vi "PPMS_Data_Recorder.vi"() -> ()   [LabVIEW 2021]
uses:
  <instrlib>/Stanford Research 830/Public/Data/Read (All Parameters).vi
  <instrlib>/Keithley 24XX/Public/Data/Read (Single Point).vi
  <instrlib>/Keithley 24XX/Keithley 24XX.lvlib
  <instrlib>/Stanford Research 830/Stanford Research 830.lvlib
panel:
  out "Phase-Vg":cluster{dbl[], dbl[]}[](graph)
  out "Leak-Vg":cluster{dbl[], dbl[]}[](graph)
  out "Signal-T":cluster{dbl[], dbl[]}[](graph)
  out "Signal-B":cluster{dbl[], dbl[]}[](graph)
  out "Signal-Vg":cluster{dbl[], dbl[]}[](graph)
  out "Voltage #3":sgl
  out "Leakage Current #3":sgl
  out "X-Value 3":dbl
  out "Theta-Value 3":dbl
  out "R-Value 3":dbl
  in  "Keithley #3 Ramp":bool
  in  "Keith#3 Comp. Lvl":dbl=1e-07
  in  "System #3 Enabled/Disabled":bool
  in  "Keithley #3":refnum<visa-resource-name>
  in  "SR830 #3":refnum<visa-resource-name>="GPIB0::10::INSTR"
  in  "SR830 #3 Input Connection":u16(ring) items=["Single-Ended Voltage", "Differential Voltage", "1 MOhm Current Gain", "100 MOhm Current Gain"]
  in  "SR830 #3\nInput Coupling":u16(ring) items=["AC", "DC"]
  in  "SR830 #3 Input \nShield Grounding":u16(ring) items=["Float", "Ground"]
  in  "SR830 #3 Input\nNotch Filter":u16(ring) items=["None", "Line Notch", "2x Line Notch", "Both Notch Filters"]
  in  "SR830 #3 Trigger Source":u16(ring) items=["Internal", "External"]
  in  "SR830 #3 Internal \nReference Frequency":dbl=17.0
  in  "SR830 #3 Detection Harm. Num.":dbl=1.0
  in  "SR830 #3 Sine \nOutput Amplitude":dbl=1.0
  in  "SR830 #3 Reference Source":u16(ring)=1 items=["External", "Internal"]
  in  "SR830 #3 Manual \nPhase":dbl
  in  "SR830 #3 \nAuto Phase":bool
  in  "SR830 #3 \nTime Constant":u16(ring)=9 items=["10 us", "30 us", "100 us", "300 us", "1 ms", "3 ms", "10 ms", "30 ms", "100 ms", "300 ms", "1 s", "3 s", "10 s", "30 s", "100 s", "300 s", "1 ks", "3 ks", "10 ks", "30 ks"]
  in  "SR830 #3 Low\nPass Filter Slope":u16(ring)=3 items=["6 dB/oct", "12 dB/oct", "18 db/oct", "24 dB/oct"]
  in  "SR830 #3\nSync Filter":bool
  in  "SR830 #3 \nDynamic Reserve":i16(ring)=1 items=["Auto Reserve"=-1, "High Reserve"=0, "Normal"=1, "Low Noise"=2]
  in  "SR830 #3\nSensitivity":i16(ring)=17 items=["Auto Gain"=-1, "2 nV/fA"=0, "5 nV/fA"=1, "10 nV/fA"=2, "20 nV/fA"=3, "50 nV/fA"=4, "100 nV/fA"=5, "200 nV/fA"=6, "500 nV/fA"=7, "1 uV/pA"=8, "2 uV/pA"=9, "5 uV/pA"=10, "10 uV/pA"=11, "20 uV/pA"=12, "50 uV/pA"=13, "100 uV/pA"=14, "200 uV/pA"=15, "500 uV/pA"=16, "1 mV/nA"=17, "2 mV/nA"=18, "5 mV/nA"=19, "10 mV/nA"=20, "20 mV/nA"=21, "50 mV/nA"=22, "100 mV/nA"=23, "200 mV/nA"=24, "500 mV/mA"=25, "1 V/uA"=26]
  in  "Keithley #3 Vg Init. (V)":dbl
  in  "Keithley #3 Vg Max (V)":dbl
  in  "Keithley #3 Vg Min (V)":dbl
  in  "Keithley #3 Vg Step (V)":dbl
  out "Voltage #2":sgl
  out "Leakage Current #2":sgl
  out "X-Value 2":dbl
  out "Theta-Value 2":dbl
  out "R-Value 2":dbl
  in  "Keithley #2 Ramp":bool
  in  "Keith#2 Comp. Lvl":dbl=1e-07
  in  "System #2 Enabled/Disabled":bool
  in  "Keithley #2":refnum<visa-resource-name>
  in  "SR830 #2":refnum<visa-resource-name>="GPIB0::10::INSTR"
  in  "SR830 #2 Input Connection":u16(ring) items=["Single-Ended Voltage", "Differential Voltage", "1 MOhm Current Gain", "100 MOhm Current Gain"]
  in  "SR830 #2\nInput Coupling":u16(ring) items=["AC", "DC"]
  in  "SR830 #2 Input \nShield Grounding":u16(ring) items=["Float", "Ground"]
  in  "SR830 #2 Input\nNotch Filter":u16(ring) items=["None", "Line Notch", "2x Line Notch", "Both Notch Filters"]
  in  "SR830 #2 Trigger Source":u16(ring) items=["Internal", "External"]
  in  "SR830 #2 Internal \nReference Frequency":dbl=17.0
  in  "SR830 #2 Detection Harm. Num.":dbl=1.0
  in  "SR830 #2 Sine \nOutput Amplitude":dbl=1.0
  in  "SR830 #2 Reference Source":u16(ring)=1 items=["External", "Internal"]
  in  "SR830 #2 Manual \nPhase":dbl
  in  "SR830 #2 \nAuto Phase":bool
  in  "SR830 #2 \nTime Constant":u16(ring)=9 items=["10 us", "30 us", "100 us", "300 us", "1 ms", "3 ms", "10 ms", "30 ms", "100 ms", "300 ms", "1 s", "3 s", "10 s", "30 s", "100 s", "300 s", "1 ks", "3 ks", "10 ks", "30 ks"]
  in  "SR830 #2 Low\nPass Filter Slope":u16(ring)=3 items=["6 dB/oct", "12 dB/oct", "18 db/oct", "24 dB/oct"]
  in  "SR830 #2\nSync Filter":bool
  in  "SR830 #2 \nDynamic Reserve":i16(ring)=1 items=["Auto Reserve"=-1, "High Reserve"=0, "Normal"=1, "Low Noise"=2]
  in  "SR830 #2\nSensitivity":i16(ring)=17 items=["Auto Gain"=-1, "2 nV/fA"=0, "5 nV/fA"=1, "10 nV/fA"=2, "20 nV/fA"=3, "50 nV/fA"=4, "100 nV/fA"=5, "200 nV/fA"=6, "500 nV/fA"=7, "1 uV/pA"=8, "2 uV/pA"=9, "5 uV/pA"=10, "10 uV/pA"=11, "20 uV/pA"=12, "50 uV/pA"=13, "100 uV/pA"=14, "200 uV/pA"=15, "500 uV/pA"=16, "1 mV/nA"=17, "2 mV/nA"=18, "5 mV/nA"=19, "10 mV/nA"=20, "20 mV/nA"=21, "50 mV/nA"=22, "100 mV/nA"=23, "200 mV/nA"=24, "500 mV/mA"=25, "1 V/uA"=26]
  in  "Keithley #2 Vg Init. (V)":dbl
  in  "Keithley #2 Vg Max (V)":dbl
  in  "Keithley #2 Vg Min (V)":dbl
  in  "Keithley #2 Vg Step (V)":dbl
  out "Temperature":dbl
  out "Field":dbl
  in  "Remote":bool
  out "Chamber Status":i32(ring) items=["ChamberUnknown"=0, "PurgedAndSealed"=1, "VentedAndSealed"=2, "Sealed"=3, "Purging"=4, "Venting"=5, "PreHiVac"=6, "HighVac"=7, "PumpContinuous"=8, "VentContinuous"=9, "ChamberFailure"=15]
  out "Measuring":bool
  out "R-Value":dbl
  out "Theta-Value":dbl
  out "X-Value":dbl
  out "Leakage Current #1":sgl
  out "Voltage #1":sgl
  in  "Keithley #1 Ramp":bool
  in  "Keith#1 Comp. Lvl":dbl=1e-07
  in  "Keithley #1 Vg Step (V)":dbl
  in  "Keithley #1 Vg Max (V)":dbl
  in  "Keithley #1 Vg Min (V)":dbl
  in  "Keithley #1 Vg Init. (V)":dbl
  in  "Keithley #1":refnum<visa-resource-name>
  in  "SR830 #1\nSensitivity":i16(ring)=17 items=["Auto Gain"=-1, "2 nV/fA"=0, "5 nV/fA"=1, "10 nV/fA"=2, "20 nV/fA"=3, "50 nV/fA"=4, "100 nV/fA"=5, "200 nV/fA"=6, "500 nV/fA"=7, "1 uV/pA"=8, "2 uV/pA"=9, "5 uV/pA"=10, "10 uV/pA"=11, "20 uV/pA"=12, "50 uV/pA"=13, "100 uV/pA"=14, "200 uV/pA"=15, "500 uV/pA"=16, "1 mV/nA"=17, "2 mV/nA"=18, "5 mV/nA"=19, "10 mV/nA"=20, "20 mV/nA"=21, "50 mV/nA"=22, "100 mV/nA"=23, "200 mV/nA"=24, "500 mV/mA"=25, "1 V/uA"=26]
  in  "SR830 #1 \nDynamic Reserve":i16(ring)=1 items=["Auto Reserve"=-1, "High Reserve"=0, "Normal"=1, "Low Noise"=2]
  in  "SR830 #1\nSync Filter":bool
  in  "SR830 #1 Low\nPass Filter Slope":u16(ring)=3 items=["6 dB/oct", "12 dB/oct", "18 db/oct", "24 dB/oct"]
  in  "SR830 #1 \nTime Constant":u16(ring)=8 items=["10 us", "30 us", "100 us", "300 us", "1 ms", "3 ms", "10 ms", "30 ms", "100 ms", "300 ms", "1 s", "3 s", "10 s", "30 s", "100 s", "300 s", "1 ks", "3 ks", "10 ks", "30 ks"]
  in  "SR830 #1 \nAuto Phase":bool
  in  "SR830 #1 Manual \nPhase":dbl
  in  "SR830 #1 Reference Source":u16(ring)=1 items=["External", "Internal"]
  in  "SR830 #1 Sine \nOutput Amplitude":dbl=1.0
  in  "SR830 #1 Detection Harm. Num.":dbl=1.0
  in  "SR830 #1 Internal \nReference Frequency":dbl=17.0
  in  "SR830 #1 Trigger Source":u16(ring) items=["Internal", "External"]
  in  "SR830 #1 Input\nNotch Filter":u16(ring) items=["None", "Line Notch", "2x Line Notch", "Both Notch Filters"]
  in  "SR830 #1 Input \nShield Grounding":u16(ring) items=["Float", "Ground"]
  in  "SR830 #1\nInput Coupling":u16(ring) items=["AC", "DC"]
  in  "SR830 #1 Input Connection":u16(ring) items=["Single-Ended Voltage", "Differential Voltage", "1 MOhm Current Gain", "100 MOhm Current Gain"]
  in  "SR830 #1":refnum<visa-resource-name>="GPIB0::10::INSTR"
  in  "System #1 Enabled/Disabled":bool
  in  "System Reset All?":bool
  in  "program_stop":bool
  out "Actual Save Path":path
  in  "<File Name>.txt (Don't add extension)":string
  in  "Data Save Path:":path=path "C:/Users/labpc/Documents/ProbeStation Users Data"
  # "Readout (Recorded)"
  # "Keithley 24XX"
  # "Ramp Settings"
  # "Current Compliance"
  # "SR830"
  # "Input Signal"
  # "Readout (Recorded)"
  # "Source / Reference"
  # "Input Filters & Sens"
  # "Readout (Recorded)"
  # "Keithley 24XX"
  # "Ramp Settings"
  # "Current Compliance"
  # "SR830"
  # "Input Signal"
  # "Readout (Recorded)"
  # "Source / Reference"
  # "Input Filters & Sens"
  # "PPMS"
  # "Readout (Recorded)"
  # "Keithley 24XX"
  # "Ramp Settings"
  # "Current Compliance"
  # "SR830"
  # "Input Signal"
  # "Readout (Recorded)"
  # "Source / Reference"
  # "Input Filters & Sens"
  # "Initialisation:\n--> Reset \n--> Instruments?"
  # "File I/O"
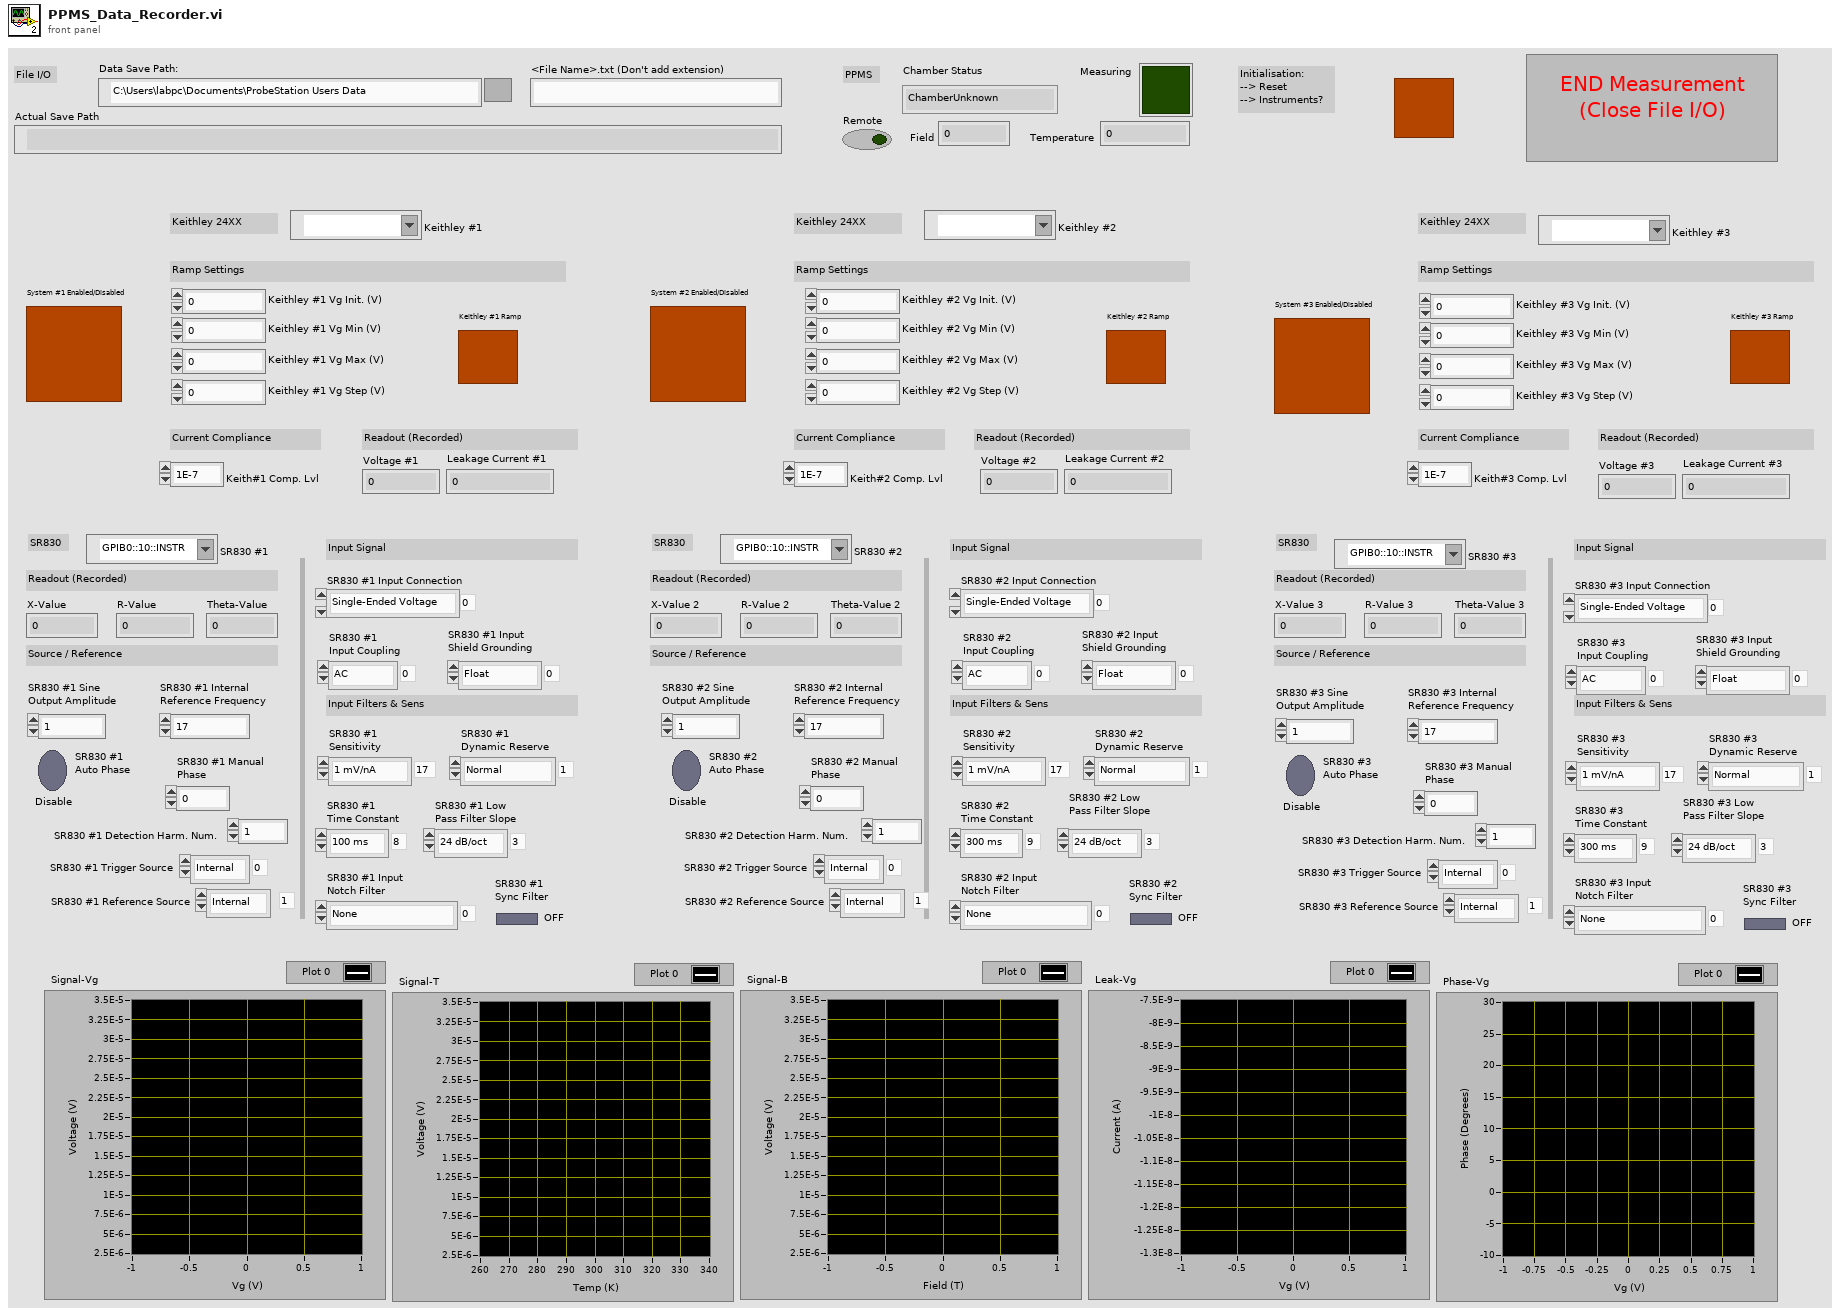
[diagram p1: front panel]
types:
  T1 = enum16{"open", "replace", "create", "open or create", "replace or create", "replace or create with confirmation"}
  T2 = cluster{"System #1 Enabled/Disabled":bool, "System #2 Enabled/Disabled":bool, "System #3 Enabled/Disabled":bool}
  T3 = cluster{"VISA resource name out":refnum<visa-resource-name>, "error out":errorcluster, "VISA resource name out":refnum<visa-resource-name>, "error out":errorcluster, "Keithley #1 Vg Init. (V)":dbl, "Keithley #1 Vg Max (V)":dbl, "Keithley #1 Vg Min (V)":dbl, "Keithley #1 Vg Step (V)":dbl, "Keith#1 Comp. Lvl":dbl}
  T4 = cluster{"Baud Rate":u32, "Parity":u16, "Data Bits":u16, "Stop Bits":u16, "Flow Control":u16}
  T5 = cluster{"VISA resource name out":refnum<visa-resource-name>, "error out":errorcluster, "VISA resource name out":refnum<visa-resource-name>, "error out":errorcluster, "Keithley #2 Vg Init. (V)":dbl, "Keithley #2 Vg Max (V)":dbl, "Keithley #2 Vg Min (V)":dbl, "Keithley #2 Vg Step (V)":dbl, "Keith#2 Comp. Lvl":dbl}
  T6 = cluster{"VISA resource name out":refnum<visa-resource-name>, "error out":errorcluster, "VISA resource name out":refnum<visa-resource-name>, "error out":errorcluster, "Keithley #3 Vg Init. (V)":dbl, "Keithley #3 Vg Max (V)":dbl, "Keithley #3 Vg Min (V)":dbl, "Keithley #3 Vg Step (V)":dbl, "Keith#3 Comp. Lvl":dbl}
  T7 = cluster{"array":dbl[][], "array":dbl[][], "array":dbl[][], "array":dbl[][]}
  T8 = cluster{"Voltage":sgl, "Current":sgl, "X-Value":dbl, "R-Value":dbl, "Theta-Value":dbl}
  T9 = enum8{"Enabled", "Disabled", "Disabled and Grayed Out"}
  T10 = cluster{"X-Value":dbl, "Y-Value":dbl, "R-Value":dbl, "Theta-Value":dbl, "Aux In 1 Value":dbl, "Aux In 2 Value":dbl, "Aux In 3 Value":dbl, "Aux In 4 Value":dbl, "Reference Frequency":dbl, "Channel 1 Display":dbl, "Channel 2 Display":dbl}
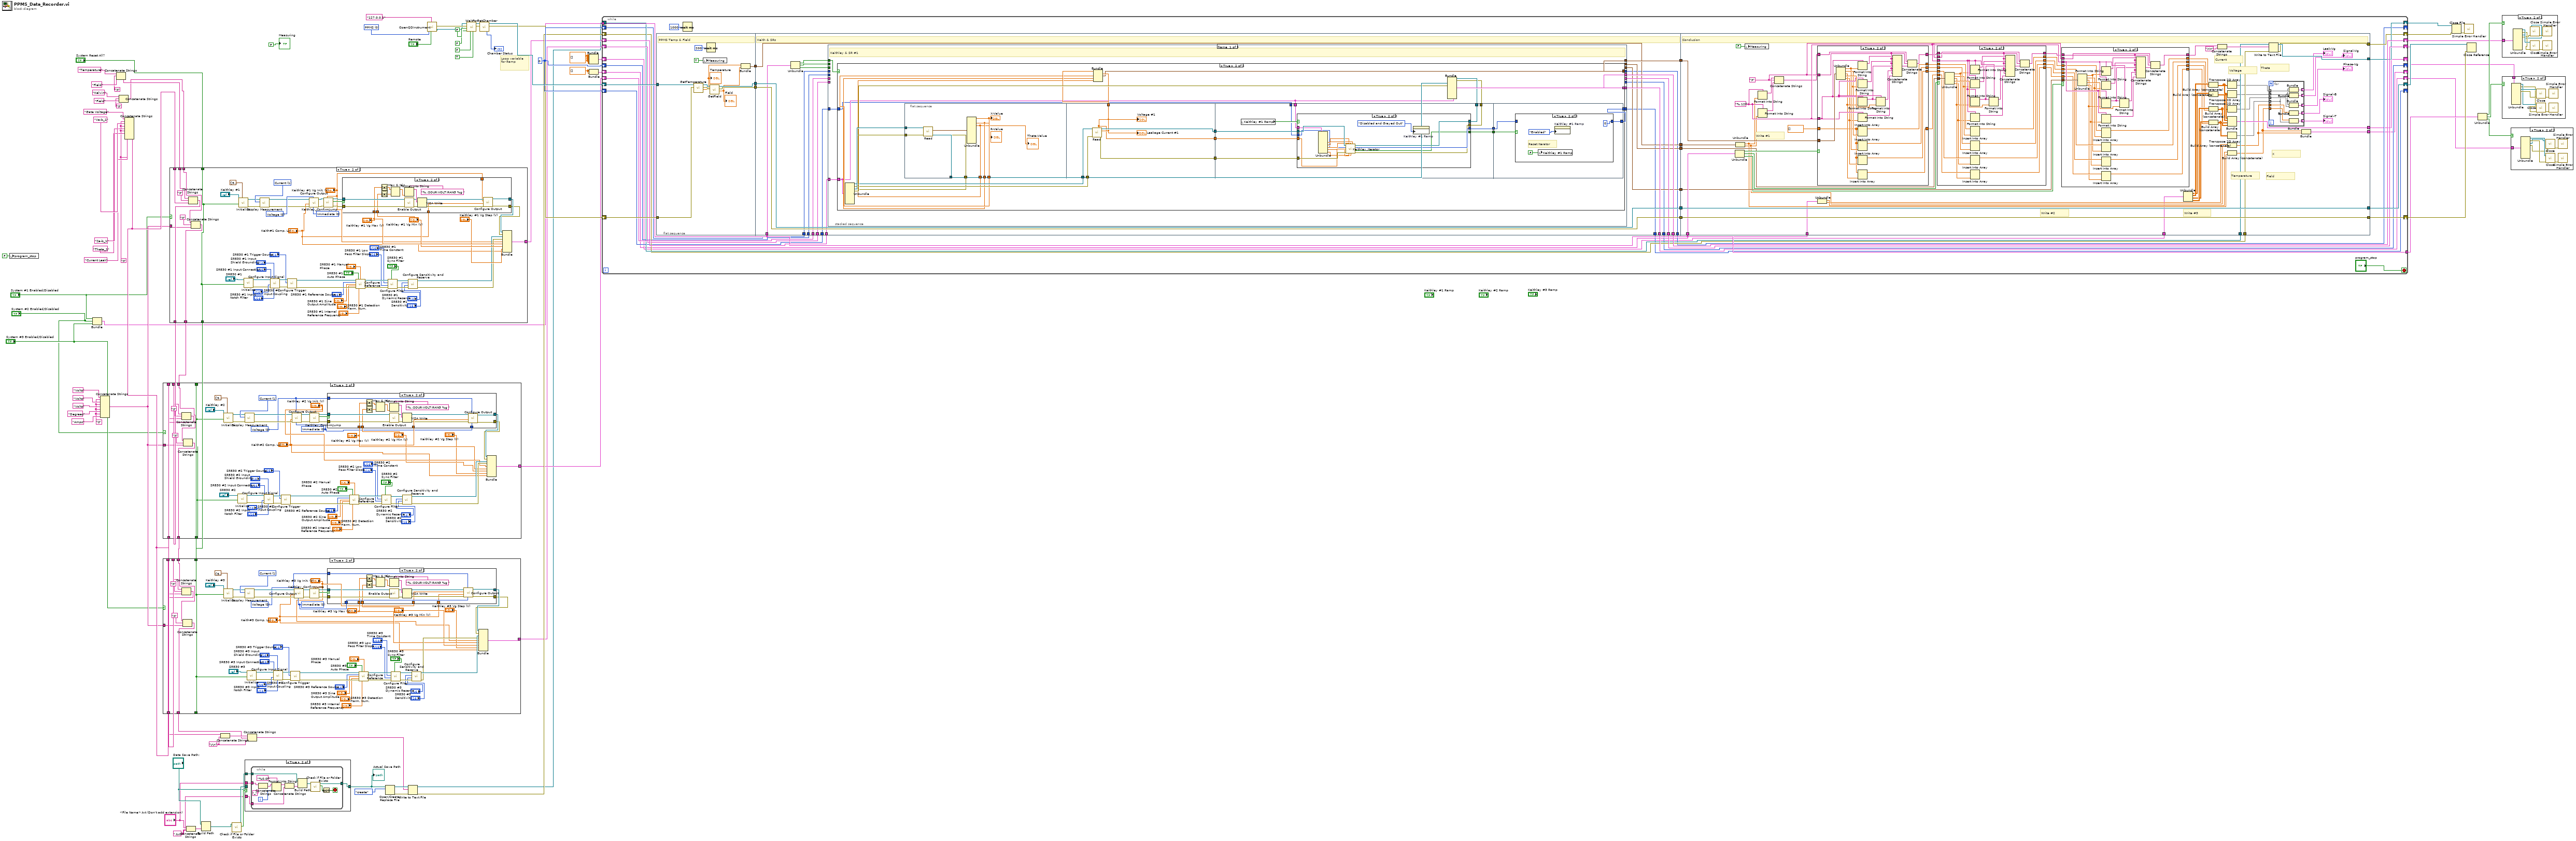
[diagram p0: block diagram]
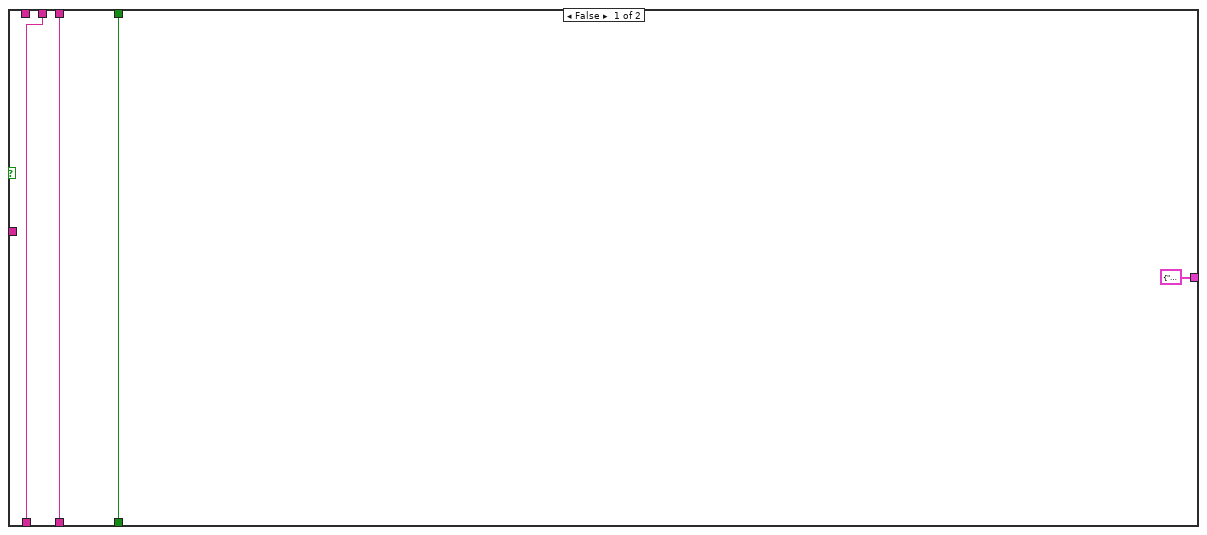
[diagram p5: hidden frame]
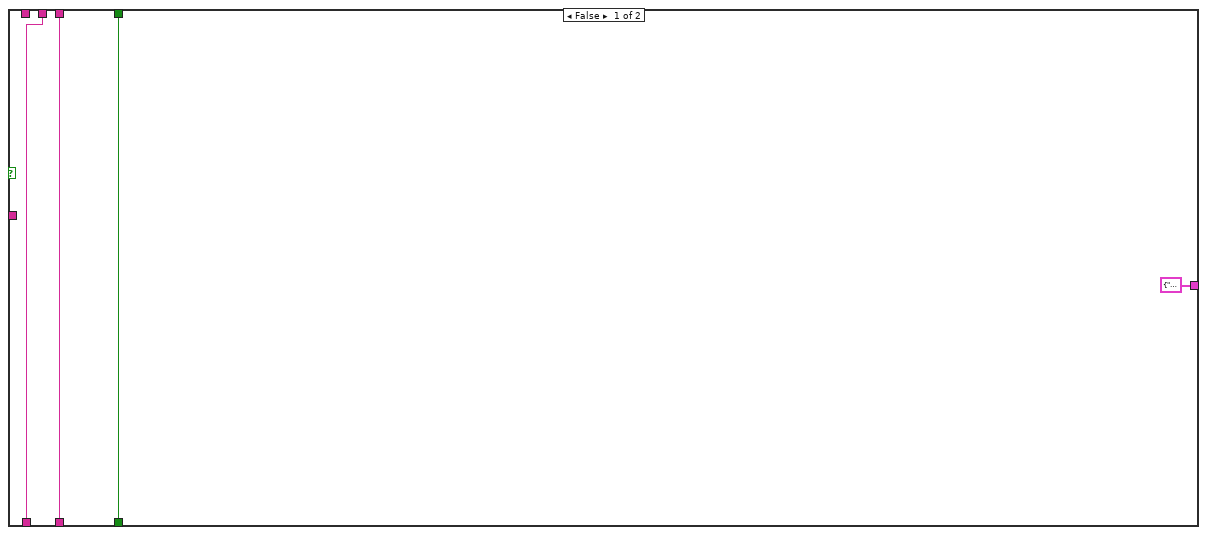
[diagram p7: hidden frame]
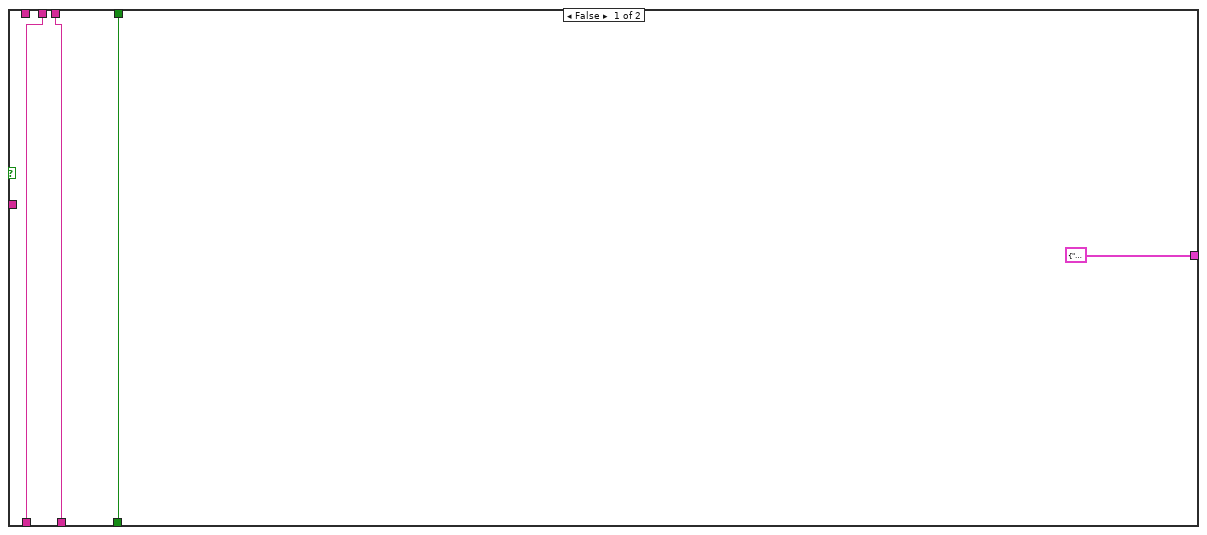
[diagram p9: hidden frame]
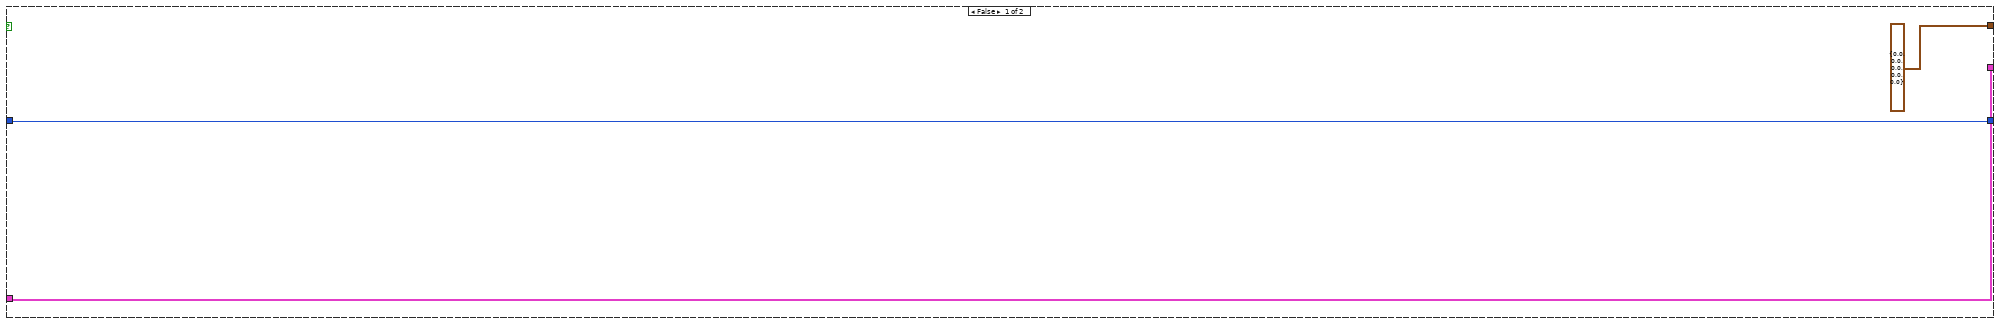
[diagram p12: hidden frame]
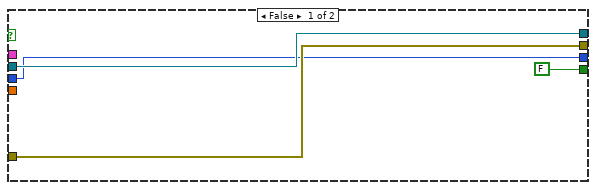
[diagram p13: hidden frame]
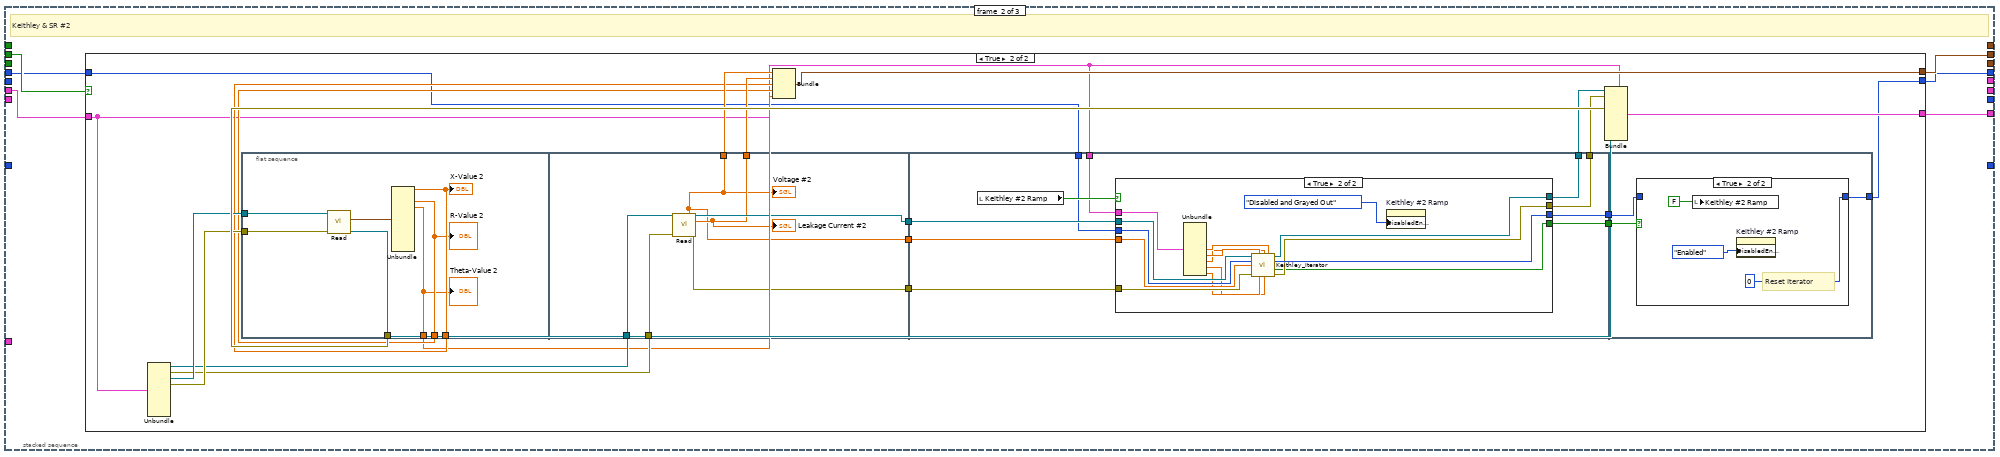
[diagram p15: hidden frame]
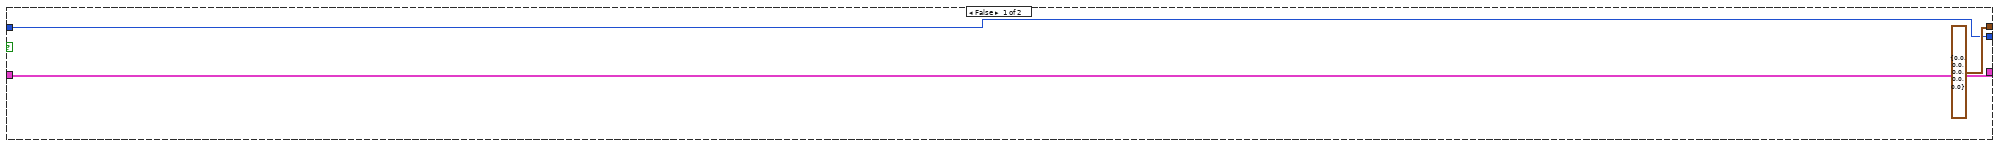
[diagram p16: hidden frame]
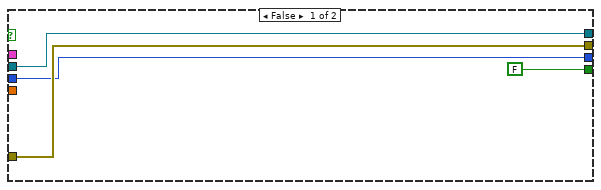
[diagram p17: hidden frame]
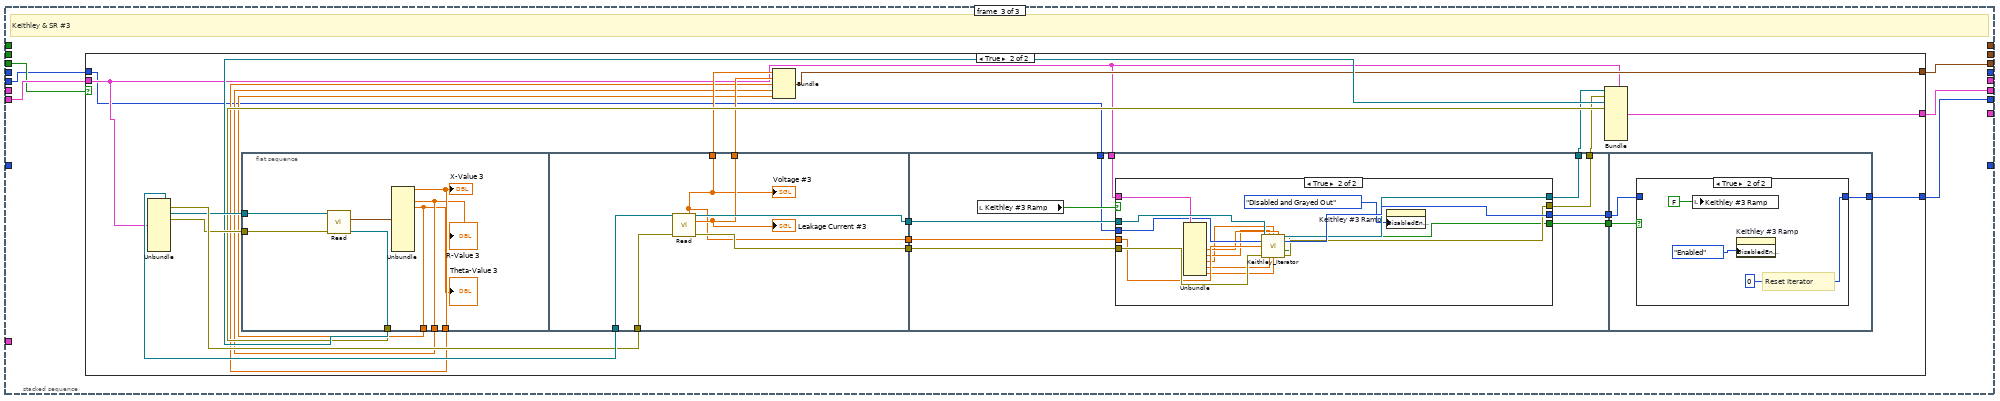
[diagram p19: hidden frame]
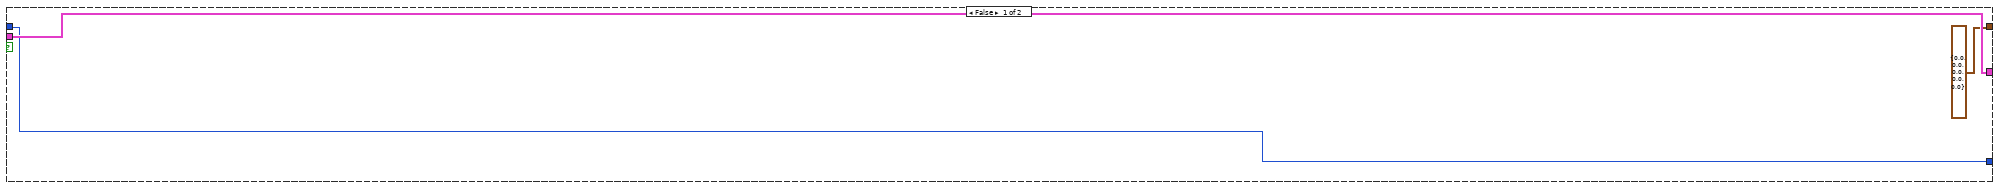
[diagram p20: hidden frame]
diagram:
  w5 = dbl[][] [] ("array")
  w7 = dbl[] [] ("array")
  w29 = 0
  w44 = "\t"
  w33 = "\r\n"
  w58 = "\t"
  w67 = 0 items=["PPMS", "VersaLab", "DynaCool", "SVSM"] ("Instrument Type")
  w70 = ".txt"
  # "Loop variable \nfor Ramp"
  n1 = local write "program_stop"(FALSE ("program_stop")) -> ()
  n2 = Bundle("System #1 Enabled/Disabled"="System #1 Enabled/Disabled", "System #2 Enabled/Disabled"="System #2 Enabled/Disabled", "System #3 Enabled/Disabled"="System #3 Enabled/Disabled") -> (w14:T2)  [unwired: 1 in]
  n3 = Concatenate Strings("Volts" ("string"), w44, "Volts" ("string"), w44, "Volts" ("string"), w44, "Degrees" ("string"), w44, "Amps" ("string")) -> (w36:string)
  n4 = Concatenate Strings("Temperature" ("string"), "\t", "Field" ("string")) -> (w57:string)
  n5 = Concatenate Strings("Kelvin" ("string"), "\t", "Field" ("string")) -> (w39:string)
  n6 = Concatenate Strings("Gate Voltage" ("string"), w58, "Va-b_1" ("string"), w58, "Za-b_1" ("string"), w58, "Theta_1" ("string"), w58, "Current Leak" ("string")) -> (w52:string)
  n7 = case shown="True" "System #1 Enabled/Disabled" {
    tunnel: w52 -> [_ w151]
    tunnel: w57 -> [w91 w149]
    tunnel: [w91 w148] -> w55
    tunnel: "System Reset All?" -> [w90 w106]
    tunnel: [w90 w106] -> w54
    tunnel: w39 -> [w89 w104]
    tunnel: [w89 w103] -> w38
    tunnel: w36 -> [_ w102]
    tunnel: [T3 {"VISA resource name out"="", "error out"={"status"=FALSE, "code"=0, "source"=""}, "VISA resource name out"="", "error out"={"status"=FALSE, "code"=0, "source"=""}, "Keithley #1 Vg Init. (V)"=0.0, "Keithley #1 Vg Max (V)"=0.0, "Keithley #1 Vg Min (V)"=0.0, "Keithley #1 Vg Step (V)"=0.0, "Keith#1 Comp. Lvl"=0.0} w94] -> w20
    frame False {
    }
    frame True {
      w112 = u16 0 items=["Immediate", "Triggered"] ("Output Type  (0: Immediate)")
      w111 = u16 0 items=["Voltage", "Current"] ("Source Mode  (0: Voltage)")
      w146 = u16 1 items=["Voltage", "Current", "Resistance"] ("Displayed Measurement (0: Voltage)")
      n8 = Concatenate Strings(w149, "\t", w151) -> (w148:string)
      n9 = Concatenate Strings(w104, "\t", w102) -> (w103:string)
      n10 = call <instrlib>:"Initialize.vi"("Serial Configuration"=T4 {"Baud Rate"=9600, "Parity"=0, "Data Bits"=8, "Stop Bits"=10, "Flow Control"=0}, "Reset (True)"=w106, "VISA resource name"="Keithley #1") -> ("error out"=w144:errorcluster, "VISA resource name out"=w145:refnum<visa-resource-name>)  [unwired: 7 in]
      n11 = call <instrlib>:"Initialize.vi"("Reset (True)"=w106, "VISA resource name"="SR830 #1") -> ("error out"=w138:errorcluster, "VISA resource name out"=w139:refnum<visa-resource-name>)  [unwired: 8 in]
      n12 = call <instrlib>:"Display Measurement.vi"("error in (no error)"=w144, "Displayed Measurement (0: Voltage)"=w146, "VISA resource name"=w145) -> ("error out"=w109:errorcluster, "VISA resource name out"=w110:refnum<visa-resource-name>)  [unwired: 7 in]
      n13 = call <instrlib>:"Configure Input Signal.vi"("Input Notch Filter (0: None)"="SR830 #1 Input\nNotch Filter", "Input Shield Grounding (0: Float)"="SR830 #1 Input \nShield Grounding", "error in (no error)"=w138, "Input Coupling (0: AC)"="SR830 #1\nInput Coupling", "Input Connection (0: Single-Ended Voltage)"="SR830 #1 Input Connection", "VISA resource name"=w139) -> ("error out"=w136:errorcluster, "VISA resource name out"=w137:refnum<visa-resource-name>)  [unwired: 4 in]
      n14 = call <instrlib>:"Configure Trigger.vi"("error in (no error)"=w136, "Trigger Source (0: Internal)"="SR830 #1 Trigger Source", "VISA resource name"=w137) -> ("error out"=w134:errorcluster, "VISA resource name out"=w135:refnum<visa-resource-name>)  [unwired: 7 in]
      n15 = call <instrlib>:"Configure Output.vi"("Output Type  (0: Immediate)"=w112, "Source Mode  (0: Voltage)"=w111, "error in (no error)"=w109, "Compliance  Level (0.1)"="Keith#1 Comp. Lvl", "VISA resource name"=w110) -> ("error out"=w107:errorcluster, "VISA resource name out"=w108:refnum<visa-resource-name>)  [unwired: 5 in]
      n16 = call "Keithley_ConfirmJump.vi"("VISA resource name in"=w108, "error in"=w107, "Gate Voltage\nInitial (V)"="Keithley #1 Vg Init. (V)") -> ("VISA resource name out"=w114:refnum<visa-resource-name>, "Voltage OK?"=w115:bool, "error out"=w113:errorcluster)  [unwired: 4 in, 1 out]
      n17 = case shown="True" w115 {
        tunnel: w114 -> [w153 w163]
        tunnel: w113 -> [w152 w162]
        tunnel: [w153 w156] -> w98
        tunnel: [w152 w157] -> w97
        tunnel: "Keithley #1 Vg Max (V)" -> [_ w161]
        tunnel: "Keithley #1 Vg Min (V)" -> [_ w160]
        tunnel: "Keithley #1 Vg Init. (V)" -> [_ w155]
        tunnel: "Keith#1 Comp. Lvl" -> [_ w154]
        frame False {
        }
        frame True {
          n18 = Absolute Value(x=w161) -> (abs(x)=w165:dbl)
          n19 = Absolute Value(x=w160) -> (abs(x)=w166:dbl)
          n20 = Max & Min(x=w165, y=w166) -> (max(x,y)=w170:dbl)  [unwired: 1 out]
          n21 = Format Into String(format string="%.;SOUR:VOLT:RANG %g ", w170) -> (resulting string=w169:string)  [unwired: 2 in, 1 out]
          n22 = call <instrlib>:"Enable Output.vi"("error in (no error)"=w162, "VISA resource name"=w163) -> ("error out"=w167:errorcluster, "VISA resource name out"=w168:refnum<visa-resource-name>)  [unwired: 8 in]
          n23 = VISA Write(VISA resource name=w168, write buffer=w169, error in (no error)=w167) -> (VISA resource name out=w159:refnum<visa-resource-name>, error out=w158:errorcluster)  [unwired: 1 out]
          n24 = call <instrlib>:"Configure Output.vi"("error in (no error)"=w158, "Compliance  Level (0.1)"=w154, "Output Level (0)"=w155, "VISA resource name"=w159) -> ("error out"=w157:errorcluster, "VISA resource name out"=w156:refnum<visa-resource-name>)  [unwired: 6 in]
        }
      }
      n25 = call <instrlib>:"Configure Reference.vi"("VISA resource name"=w135, "Auto Phase (T: Enabled)"="SR830 #1 \nAuto Phase", "Manual Phase (0 Degree)"="SR830 #1 Manual \nPhase", "Reference Source (1: Internal)"="SR830 #1 Reference Source", "Sine Output Amplitude (1 V)"="SR830 #1 Sine \nOutput Amplitude", "Detection Harmonic Number (1)"="SR830 #1 Detection Harm. Num.", "error in (no error)"=w134, "Internal Reference Frequency (1000 Hz)"="SR830 #1 Internal \nReference Frequency") -> ("VISA resource name out"=w132:refnum<visa-resource-name>, "error out"=w133:errorcluster)  [unwired: 6 in]
      n26 = call <instrlib>:"Configure Filter.vi"("Enable Sync Filter (F: Disable)"="SR830 #1\nSync Filter", "error in (no error)"=w133, "Low Pass Filter Slope (1: 12dB/oct)"="SR830 #1 Low\nPass Filter Slope", "Time Constant (8: 100ms)"="SR830 #1 \nTime Constant", "VISA resource name"=w132) -> ("error out"=w118:errorcluster, "VISA resource name out"=w119:refnum<visa-resource-name>)  [unwired: 5 in]
      n27 = call <instrlib>:"Configure Sensitivity and Reserve.vi"("error in (no error)"=w118, "Sensitivity (-1: Auto gain)"="SR830 #1\nSensitivity", "Dynamic Reserve (-1: Auto Reserve)"="SR830 #1 \nDynamic Reserve", "VISA resource name"=w119) -> ("error out"=w95:errorcluster, "VISA resource name out"=w96:refnum<visa-resource-name>)  [unwired: 6 in]
      n28 = Bundle("VISA resource name out"=w98, "error out"=w97, "VISA resource name out"=w96, "error out"=w95, "Keithley #1 Vg Init. (V)"="Keithley #1 Vg Init. (V)", "Keithley #1 Vg Max (V)"="Keithley #1 Vg Max (V)", "Keithley #1 Vg Min (V)"="Keithley #1 Vg Min (V)", "Keithley #1 Vg Step (V)"="Keithley #1 Vg Step (V)", "Keith#1 Comp. Lvl"="Keith#1 Comp. Lvl") -> (w94:T3)  [unwired: 1 in]
    }
  }
  n29 = case shown="True" "System #2 Enabled/Disabled" {
    tunnel: w52 -> [_ w234]
    tunnel: w55 -> [w174 w232]
    tunnel: [w174 w231] -> w53
    tunnel: w54 -> [w173 w195]
    tunnel: [w173 w195] -> w51
    tunnel: w38 -> [w172 w193]
    tunnel: [w172 w192] -> w37
    tunnel: w36 -> [_ w191]
    tunnel: [T5 {"VISA resource name out"="", "error out"={"status"=FALSE, "code"=0, "source"=""}, "VISA resource name out"="", "error out"={"status"=FALSE, "code"=0, "source"=""}, "Keithley #2 Vg Init. (V)"=0.0, "Keithley #2 Vg Max (V)"=0.0, "Keithley #2 Vg Min (V)"=0.0, "Keithley #2 Vg Step (V)"=0.0, "Keith#2 Comp. Lvl"=0.0} w182] -> w19
    frame False {
    }
    frame True {
      w175 = u16 0 items=["Immediate", "Triggered"] ("Output Type  (0: Immediate)")
      w176 = u16 0 items=["Voltage", "Current"] ("Source Mode  (0: Voltage)")
      w229 = u16 1 items=["Voltage", "Current", "Resistance"] ("Displayed Measurement (0: Voltage)")
      n30 = Concatenate Strings(w232, "\t", w234) -> (w231:string)
      n31 = Concatenate Strings(w193, "\t", w191) -> (w192:string)
      n32 = call <instrlib>:"Initialize.vi"("Serial Configuration"=T4 {"Baud Rate"=9600, "Parity"=0, "Data Bits"=8, "Stop Bits"=10, "Flow Control"=0}, "Reset (True)"=w195, "VISA resource name"="Keithley #2") -> ("error out"=w227:errorcluster, "VISA resource name out"=w228:refnum<visa-resource-name>)  [unwired: 7 in]
      n33 = call <instrlib>:"Initialize.vi"("Reset (True)"=w195, "VISA resource name"="SR830 #2") -> ("error out"=w221:errorcluster, "VISA resource name out"=w222:refnum<visa-resource-name>)  [unwired: 8 in]
      n34 = call <instrlib>:"Display Measurement.vi"("error in (no error)"=w227, "Displayed Measurement (0: Voltage)"=w229, "VISA resource name"=w228) -> ("error out"=w180:errorcluster, "VISA resource name out"=w181:refnum<visa-resource-name>)  [unwired: 7 in]
      n35 = call <instrlib>:"Configure Input Signal.vi"("Input Notch Filter (0: None)"="SR830 #2 Input\nNotch Filter", "Input Shield Grounding (0: Float)"="SR830 #2 Input \nShield Grounding", "error in (no error)"=w221, "Input Coupling (0: AC)"="SR830 #2\nInput Coupling", "Input Connection (0: Single-Ended Voltage)"="SR830 #2 Input Connection", "VISA resource name"=w222) -> ("error out"=w219:errorcluster, "VISA resource name out"=w220:refnum<visa-resource-name>)  [unwired: 4 in]
      n36 = call <instrlib>:"Configure Trigger.vi"("error in (no error)"=w219, "Trigger Source (0: Internal)"="SR830 #2 Trigger Source", "VISA resource name"=w220) -> ("error out"=w217:errorcluster, "VISA resource name out"=w218:refnum<visa-resource-name>)  [unwired: 7 in]
      n37 = call <instrlib>:"Configure Output.vi"("Output Type  (0: Immediate)"=w175, "Source Mode  (0: Voltage)"=w176, "error in (no error)"=w180, "Compliance  Level (0.1)"="Keith#2 Comp. Lvl", "VISA resource name"=w181) -> ("error out"=w178:errorcluster, "VISA resource name out"=w177:refnum<visa-resource-name>)  [unwired: 5 in]
      n38 = call "Keithley_ConfirmJump.vi"("VISA resource name in"=w177, "error in"=w178, "Gate Voltage\nInitial (V)"="Keithley #2 Vg Init. (V)") -> ("VISA resource name out"=w197:refnum<visa-resource-name>, "Voltage OK?"=w198:bool, "error out"=w196:errorcluster)  [unwired: 4 in, 1 out]
      n39 = case shown="True" w198 {
        tunnel: w197 -> [w236 w247]
        tunnel: w196 -> [w235 w246]
        tunnel: [w236 w238] -> w190
        tunnel: [w235 w237] -> w189
        tunnel: "Keithley #2 Vg Max (V)" -> [_ w245]
        tunnel: "Keithley #2 Vg Min (V)" -> [_ w244]
        tunnel: w175 -> [_ w243]
        tunnel: w176 -> [_ w242]
        tunnel: "Keith#2 Comp. Lvl" -> [_ w241]
        frame False {
        }
        frame True {
          n40 = Absolute Value(x=w245) -> (abs(x)=w249:dbl)
          n41 = Absolute Value(x=w244) -> (abs(x)=w250:dbl)
          n42 = Max & Min(x=w249, y=w250) -> (max(x,y)=w254:dbl)  [unwired: 1 out]
          n43 = Format Into String(format string="%.;SOUR:VOLT:RANG %g ", w254) -> (resulting string=w253:string)  [unwired: 2 in, 1 out]
          n44 = call <instrlib>:"Enable Output.vi"("error in (no error)"=w246, "VISA resource name"=w247) -> ("error out"=w251:errorcluster, "VISA resource name out"=w252:refnum<visa-resource-name>)  [unwired: 8 in]
          n45 = VISA Write(VISA resource name=w252, write buffer=w253, error in (no error)=w251) -> (VISA resource name out=w240:refnum<visa-resource-name>, error out=w239:errorcluster)  [unwired: 1 out]
          n46 = call <instrlib>:"Configure Output.vi"("Output Type  (0: Immediate)"=w243, "Source Mode  (0: Voltage)"=w242, "error in (no error)"=w239, "Compliance  Level (0.1)"=w241, "VISA resource name"=w240) -> ("error out"=w237:errorcluster, "VISA resource name out"=w238:refnum<visa-resource-name>)  [unwired: 5 in]
        }
      }
      n47 = call <instrlib>:"Configure Reference.vi"("VISA resource name"=w218, "Auto Phase (T: Enabled)"="SR830 #2 \nAuto Phase", "Manual Phase (0 Degree)"="SR830 #2 Manual \nPhase", "Reference Source (1: Internal)"="SR830 #2 Reference Source", "Sine Output Amplitude (1 V)"="SR830 #2 Sine \nOutput Amplitude", "Detection Harmonic Number (1)"="SR830 #2 Detection Harm. Num.", "error in (no error)"=w217, "Internal Reference Frequency (1000 Hz)"="SR830 #2 Internal \nReference Frequency") -> ("VISA resource name out"=w215:refnum<visa-resource-name>, "error out"=w216:errorcluster)  [unwired: 6 in]
      n48 = call <instrlib>:"Configure Filter.vi"("Enable Sync Filter (F: Disable)"="SR830 #2\nSync Filter", "error in (no error)"=w216, "Low Pass Filter Slope (1: 12dB/oct)"="SR830 #2 Low\nPass Filter Slope", "Time Constant (8: 100ms)"="SR830 #2 \nTime Constant", "VISA resource name"=w215) -> ("error out"=w201:errorcluster, "VISA resource name out"=w202:refnum<visa-resource-name>)  [unwired: 5 in]
      n49 = call <instrlib>:"Configure Sensitivity and Reserve.vi"("error in (no error)"=w201, "Sensitivity (-1: Auto gain)"="SR830 #2\nSensitivity", "Dynamic Reserve (-1: Auto Reserve)"="SR830 #2 \nDynamic Reserve", "VISA resource name"=w202) -> ("error out"=w187:errorcluster, "VISA resource name out"=w188:refnum<visa-resource-name>)  [unwired: 6 in]
      n50 = Bundle("VISA resource name out"=w190, "error out"=w189, "VISA resource name out"=w188, "error out"=w187, "Keithley #2 Vg Init. (V)"="Keithley #2 Vg Init. (V)", "Keithley #2 Vg Max (V)"="Keithley #2 Vg Max (V)", "Keithley #2 Vg Min (V)"="Keithley #2 Vg Min (V)", "Keithley #2 Vg Step (V)"="Keithley #2 Vg Step (V)", "Keith#2 Comp. Lvl"="Keith#2 Comp. Lvl") -> (w182:T5)  [unwired: 1 in]
    }
  }
  n51 = case shown="True" "System #3 Enabled/Disabled" {
    tunnel: w52 -> [_ w318]
    tunnel: w53 -> [w258 w316]
    tunnel: [w258 w315] -> w50
    tunnel: w51 -> [w257 w275]
    tunnel: [w257 w275] -> _
    tunnel: w37 -> [w256 w273]
    tunnel: w36 -> [_ w272]
    tunnel: [w256 w271] -> w31
    tunnel: [T6 {"VISA resource name out"="", "error out"={"status"=FALSE, "code"=0, "source"=""}, "VISA resource name out"="", "error out"={"status"=FALSE, "code"=0, "source"=""}, "Keithley #3 Vg Init. (V)"=0.0, "Keithley #3 Vg Max (V)"=0.0, "Keithley #3 Vg Min (V)"=0.0, "Keithley #3 Vg Step (V)"=0.0, "Keith#3 Comp. Lvl"=0.0} w263] -> w18
    frame False {
    }
    frame True {
      w261 = u16 0 items=["Immediate", "Triggered"] ("Output Type  (0: Immediate)")
      w262 = u16 0 items=["Voltage", "Current"] ("Source Mode  (0: Voltage)")
      w313 = u16 1 items=["Voltage", "Current", "Resistance"] ("Displayed Measurement (0: Voltage)")
      n52 = Concatenate Strings(w316, "\t", w318) -> (w315:string)
      n53 = Concatenate Strings(w273, "\t", w272) -> (w271:string)
      n54 = call <instrlib>:"Initialize.vi"("Serial Configuration"=T4 {"Baud Rate"=9600, "Parity"=0, "Data Bits"=8, "Stop Bits"=10, "Flow Control"=0}, "Reset (True)"=w275, "VISA resource name"="Keithley #3") -> ("error out"=w311:errorcluster, "VISA resource name out"=w312:refnum<visa-resource-name>)  [unwired: 7 in]
      n55 = call <instrlib>:"Display Measurement.vi"("error in (no error)"=w311, "Displayed Measurement (0: Voltage)"=w313, "VISA resource name"=w312) -> ("error out"=w278:errorcluster, "VISA resource name out"=w279:refnum<visa-resource-name>)  [unwired: 7 in]
      n56 = call <instrlib>:"Initialize.vi"("Reset (True)"=w275, "VISA resource name"="SR830 #3") -> ("error out"=w305:errorcluster, "VISA resource name out"=w306:refnum<visa-resource-name>)  [unwired: 8 in]
      n57 = call <instrlib>:"Configure Input Signal.vi"("Input Notch Filter (0: None)"="SR830 #3 Input\nNotch Filter", "Input Shield Grounding (0: Float)"="SR830 #3 Input \nShield Grounding", "error in (no error)"=w305, "Input Coupling (0: AC)"="SR830 #3\nInput Coupling", "Input Connection (0: Single-Ended Voltage)"="SR830 #3 Input Connection", "VISA resource name"=w306) -> ("error out"=w303:errorcluster, "VISA resource name out"=w304:refnum<visa-resource-name>)  [unwired: 4 in]
      n58 = call <instrlib>:"Configure Trigger.vi"("error in (no error)"=w303, "Trigger Source (0: Internal)"="SR830 #3 Trigger Source", "VISA resource name"=w304) -> ("error out"=w301:errorcluster, "VISA resource name out"=w302:refnum<visa-resource-name>)  [unwired: 7 in]
      n59 = call <instrlib>:"Configure Output.vi"("Output Type  (0: Immediate)"=w261, "Source Mode  (0: Voltage)"=w262, "error in (no error)"=w278, "Compliance  Level (0.1)"="Keith#3 Comp. Lvl", "VISA resource name"=w279) -> ("error out"=w276:errorcluster, "VISA resource name out"=w277:refnum<visa-resource-name>)  [unwired: 5 in]
      n60 = call "Keithley_ConfirmJump.vi"("VISA resource name in"=w277, "error in"=w276, "Gate Voltage\nInitial (V)"="Keithley #3 Vg Init. (V)") -> ("VISA resource name out"=w281:refnum<visa-resource-name>, "Voltage OK?"=w282:bool, "error out"=w280:errorcluster)  [unwired: 4 in, 1 out]
      n61 = case shown="True" w282 {
        tunnel: w281 -> [w320 w332]
        tunnel: w280 -> [w319 w331]
        tunnel: [w320 w325] -> w270
        tunnel: [w319 w326] -> w269
        tunnel: "Keithley #3 Vg Max (V)" -> [_ w330]
        tunnel: "Keithley #3 Vg Min (V)" -> [_ w329]
        tunnel: w262 -> [_ w324]
        tunnel: w261 -> [_ w323]
        tunnel: "Keithley #3 Vg Init. (V)" -> [_ w322]
        tunnel: "Keith#3 Comp. Lvl" -> [_ w321]
        frame False {
        }
        frame True {
          n62 = Absolute Value(x=w330) -> (abs(x)=w334:dbl)
          n63 = Absolute Value(x=w329) -> (abs(x)=w335:dbl)
          n64 = Max & Min(x=w334, y=w335) -> (max(x,y)=w339:dbl)  [unwired: 1 out]
          n65 = Format Into String(format string="%.;SOUR:VOLT:RANG %g ", w339) -> (resulting string=w338:string)  [unwired: 2 in, 1 out]
          n66 = call <instrlib>:"Enable Output.vi"("error in (no error)"=w331, "VISA resource name"=w332) -> ("error out"=w336:errorcluster, "VISA resource name out"=w337:refnum<visa-resource-name>)  [unwired: 8 in]
          n67 = VISA Write(VISA resource name=w337, write buffer=w338, error in (no error)=w336) -> (VISA resource name out=w328:refnum<visa-resource-name>, error out=w327:errorcluster)  [unwired: 1 out]
          n68 = call <instrlib>:"Configure Output.vi"("Output Type  (0: Immediate)"=w323, "Source Mode  (0: Voltage)"=w324, "error in (no error)"=w327, "Compliance  Level (0.1)"=w321, "Output Level (0)"=w322, "VISA resource name"=w328) -> ("error out"=w326:errorcluster, "VISA resource name out"=w325:refnum<visa-resource-name>)  [unwired: 4 in]
        }
      }
      n69 = call <instrlib>:"Configure Reference.vi"("VISA resource name"=w302, "Auto Phase (T: Enabled)"="SR830 #3 \nAuto Phase", "Manual Phase (0 Degree)"="SR830 #3 Manual \nPhase", "Reference Source (1: Internal)"="SR830 #3 Reference Source", "Sine Output Amplitude (1 V)"="SR830 #3 Sine \nOutput Amplitude", "Detection Harmonic Number (1)"="SR830 #3 Detection Harm. Num.", "error in (no error)"=w301, "Internal Reference Frequency (1000 Hz)"="SR830 #3 Internal \nReference Frequency") -> ("VISA resource name out"=w299:refnum<visa-resource-name>, "error out"=w300:errorcluster)  [unwired: 6 in]
      n70 = call <instrlib>:"Configure Filter.vi"("Enable Sync Filter (F: Disable)"="SR830 #3\nSync Filter", "error in (no error)"=w300, "Low Pass Filter Slope (1: 12dB/oct)"="SR830 #3 Low\nPass Filter Slope", "Time Constant (8: 100ms)"="SR830 #3 \nTime Constant", "VISA resource name"=w299) -> ("error out"=w285:errorcluster, "VISA resource name out"=w286:refnum<visa-resource-name>)  [unwired: 5 in]
      n71 = call <instrlib>:"Configure Sensitivity and Reserve.vi"("error in (no error)"=w285, "Sensitivity (-1: Auto gain)"="SR830 #3\nSensitivity", "Dynamic Reserve (-1: Auto Reserve)"="SR830 #3 \nDynamic Reserve", "VISA resource name"=w286) -> ("error out"=w267:errorcluster, "VISA resource name out"=w268:refnum<visa-resource-name>)  [unwired: 6 in]
      n72 = Bundle("VISA resource name out"=w270, "error out"=w269, "VISA resource name out"=w268, "error out"=w267, "Keithley #3 Vg Init. (V)"="Keithley #3 Vg Init. (V)", "Keithley #3 Vg Max (V)"="Keithley #3 Vg Max (V)", "Keithley #3 Vg Min (V)"="Keithley #3 Vg Min (V)", "Keithley #3 Vg Step (V)"="Keithley #3 Vg Step (V)", "Keith#3 Comp. Lvl"="Keith#3 Comp. Lvl") -> (w263:T6)  [unwired: 1 in]
    }
  }
  n73 = Concatenate Strings("<File Name>.txt (Don't add extension)", w70) -> (w76:string)
  n74 = Build Path(base path="Data Save Path:", name or relative path=w76) -> (appended path=w75:path)
  n75 = Concatenate Strings(w50, w33) -> (w32:string)
  n76 = call <vilib>:"Check if File or Folder Exists.vi"("path"=w75) -> ("file or folder exists?"=w74:bool, "dup path"=w73:path)  [unwired: 8 in, 1 out]
  n77 = case shown="True" w74 {
    tunnel: [w340 w341] -> w68
    tunnel: w73 -> [w340 _]
    tunnel: "Data Save Path:" -> [_ w342]
    tunnel: "<File Name>.txt (Don't add extension)" -> [_ w344]
    tunnel: w70 -> [_ w343]
    frame False {
    }
    frame True {
      n78 = while {
        tunnel: w344 -> [w347]
        tunnel: w343 -> [w352]
        tunnel: w342 -> [w350]
        tunnel: [w348] -> w341
        i -> [w354]
        stop <- w356 stop-if-true
        n79 = Concatenate Strings(w347, "_" ("string")) -> (w346:string)
        n80 = Format Into String(format string="%0.0f", initial string=w346, w354) -> (resulting string=w353:string)  [unwired: 1 in, 1 out]
        n81 = Concatenate Strings(w353, w352) -> (w351:string)
        n82 = Build Path(base path=w350, name or relative path=w351) -> (appended path=w349:path)
        n83 = call <vilib>:"Check if File or Folder Exists.vi"("path"=w349) -> ("file or folder exists?"=w357:bool, "dup path"=w348:path)  [unwired: 8 in, 1 out]
        n84 = Not(x=w357) -> (.not. x?=w356:bool)
      }
    }
  }
  "Actual Save Path" <- w68
  n85 = Concatenate Strings(w32, w31, w33) -> (w30:string)
  n86 = Open/Create/Replace File(file path (use dialog)=w68, operation (0:open)=T1."create") -> (refnum out=w35:refnum<file>, error out=w34:errorcluster)  [unwired: 4 in, 1 out]
  n87 = Write to Text File(file (use dialog)=w35, text=w30, error in=w34) -> (refnum out=w9:refnum<file>, error out=w25:errorcluster)  [unwired: 1 in, 1 out]
  n88 = call "OpenQDInstrument.vi"("Remote"="Remote", "IP Address"="127.0.0.1", "Instrument Type"=w67) -> ("error out"=w79:errorcluster, "Instrument Ref"=w78:refnum<k24>)  [unwired: 5 in]
  n89 = call "WaitFor.vi"("Wait For Chamber"=TRUE ("WaitForChamber"), "Wait For Position"=FALSE ("WaitForPosition"), "Wait For Field"=FALSE ("WaitForField"), "Wait For Temperature"=FALSE ("WaitForTemperature"), "error in (no error)"=w79, "Instrument Ref In"=w78) -> ("error out"=w83:errorcluster, "Instrument Ref Out"=w82:refnum<k24>)  [unwired: 4 in]
  n90 = call "GetChamber.vi"("error in (no error)"=w83, "Instrument Ref In"=w82) -> ("Chamber\nStatus"=→"Chamber Status":i32, "error out"=w27:errorcluster, "Instrument Ref Out"=w28:refnum<k24>)  [unwired: 2 in, 1 out]
  n91 = Bundle("array"=w5, "array"=w5, "array"=w5, "array"=w5) -> (w8:T7)  [unwired: 1 in]
  n92 = Bundle("array"=w7, "array"=w7) -> (w6:cluster{"array":dbl[], "array":dbl[]})  [unwired: 1 in]
  n93 = while {
    shift-right: [w365] -> _
    shift-left: w29 -> [w367]
    shift-right: [w364] -> _
    shift-left: w29 -> [w366]
    shift-right: [w362] -> _
    shift-left: w29 -> [w363]
    shift-right: [w388] -> w23
    shift-left: w28 -> [w391]
    shift-right: [w386] -> w24
    shift-left: w27 -> [w390]
    shift-right: [w370] -> w22
    shift-left: w9 -> [w371]
    shift-right: [w368] -> w21
    shift-left: w25 -> [w369]
    shift-right: [w380] -> w4
    shift-left: w20 -> [w383]
    shift-right: [w379] -> w2
    shift-left: w19 -> [w382]
    shift-right: [w378] -> w3
    shift-left: w18 -> [w381]
    tunnel: w14 -> [w372]
    tunnel: [w372] -> w13
    shift-right: [w358] -> _
    shift-left: w8 -> [w361]
    shift-right: [w359] -> _
    shift-left: w6 -> [w360]
    stop <- "program_stop" stop-if-true
    n94 = flat-sequence {
      tunnel: w391 -> [w400]
      tunnel: w390 -> [w399]
      tunnel: [w398] -> w389
      tunnel: [w397] -> w387
      tunnel: [w394] -> w373
      tunnel: [w426] -> w385
      tunnel: w389 -> [w426]
      tunnel: [w425] -> w384
      tunnel: w387 -> [w425]
      tunnel: w383 -> [w424]
      tunnel: w382 -> [w423]
      tunnel: w381 -> [w422]
      tunnel: [w421] -> w380
      tunnel: [w420] -> w379
      tunnel: [w419] -> w378
      tunnel: w372 -> [w418]
      tunnel: [w414] -> w377
      tunnel: [w413] -> w376
      tunnel: [w412] -> w375
      tunnel: [w411] -> w374
      tunnel: w373 -> [w411]
      tunnel: w367 -> [w410]
      tunnel: w366 -> [w409]
      tunnel: [w408] -> w365
      tunnel: [w407] -> w364
      tunnel: w363 -> [w406]
      tunnel: [w405] -> w362
      tunnel: [w736] -> w388
      tunnel: w385 -> [w736]
      tunnel: [w735] -> w386
      tunnel: w384 -> [w735]
      tunnel: w377 -> [w732]
      tunnel: w376 -> [w730]
      tunnel: w375 -> [w729]
      tunnel: w374 -> [w731]
      tunnel: w372 -> [w734]
      tunnel: w371 -> [w716]
      tunnel: w369 -> [w714]
      tunnel: [w715] -> w370
      tunnel: [w713] -> w368
      tunnel: w361 -> [w702]
      tunnel: w360 -> [w708]
      tunnel: [w707] -> w359
      tunnel: [w701] -> w358
      frame #0 {
        # "PPMS Temp & Field"
        n95 = call "GetTemperature.vi"("error in (no error)"=w399, "Instrument Ref In"=w400) -> ("Temperature"=w396:dbl, "error out"=w403:errorcluster, "Instrument Ref Out"=w404:refnum<k24>)  [unwired: 3 in, 2 out]
        "Temperature" <- w396
        n96 = local write "Measuring"(TRUE ("Measuring")) -> ()
        n97 = Wait (ms)(milliseconds to wait=u32 200) -> ()  [unwired: 1 out]
        n98 = call "GetField.vi"("error in (no error)"=w403, "Instrument Ref In"=w404) -> ("Field"=w395:dbl, "error out"=w397:errorcluster, "Instrument Ref Out"=w398:refnum<k24>)  [unwired: 3 in, 2 out]
        "Field" <- w395
        n99 = Bundle("Temperature"=w396, "Field"=w395) -> (w394:cluster{"Temperature":dbl, "Field":dbl})  [unwired: 1 in]
      }
      frame #1 {
        # "Keith & SRs"
        n100 = Unbundle(w418) -> ("System #1 Enabled/Disabled"=w417:bool, "System #2 Enabled/Disabled"=w416:bool, "System #3 Enabled/Disabled"=w415:bool)
        n101 = stacked-sequence {
          tunnel: w424 -> [w432 _ _]
          tunnel: w423 -> [_ w513 _]
          tunnel: w422 -> [_ _ w595]
          tunnel: [w431 _ _] -> w421
          tunnel: [_ w514 _] -> w420
          tunnel: [_ _ w596] -> w419
          tunnel: w417 -> [w430 _ _]
          tunnel: w416 -> [_ w512 _]
          tunnel: w415 -> [_ _ w594]
          tunnel: [w429 _ _] -> w414
          tunnel: [_ w511 _] -> w413
          tunnel: [_ _ w593] -> w412
          tunnel: w410 -> [w428 _ _]
          tunnel: w409 -> [_ w510 _]
          tunnel: [w427 _ _] -> w408
          tunnel: [_ w509 _] -> w407
          tunnel: w406 -> [_ _ w592]
          tunnel: [_ _ w591] -> w405
          frame #0 {
            # "Keithley & SR #1"
            n102 = case shown="True" w430 {
              tunnel: w432 -> [w435 w438]
              tunnel: [w435 w453] -> w431
              tunnel: [T8 {"Voltage"=0.0, "Current"=0.0, "X-Value"=0.0, "R-Value"=0.0, "Theta-Value"=0.0} w439] -> w429
              tunnel: w428 -> [w433 w437]
              tunnel: [w433 w436] -> w427
              frame False {
              }
              frame True {
                n103 = Unbundle(w438) -> ("VISA resource name out"=w450:refnum<visa-resource-name>, "error out"=w449:errorcluster, "VISA resource name out"=w452:refnum<visa-resource-name>, "error out"=w451:errorcluster)  [unwired: 5 out]
                n104 = flat-sequence {
                  tunnel: [w466] -> w446
                  tunnel: [w465] -> w445
                  tunnel: [w463] -> w442
                  tunnel: [w462] -> w441
                  tunnel: [w461] -> w440
                  tunnel: w452 -> [w460]
                  tunnel: w451 -> [w459]
                  tunnel: [w472] -> w458
                  tunnel: [w471] -> w457
                  tunnel: [w467] -> w456
                  tunnel: [w470] -> w443
                  tunnel: w450 -> [w469]
                  tunnel: w449 -> [w468]
                  tunnel: [w467] -> w444
                  tunnel: w458 -> [w481]
                  tunnel: w457 -> [w480]
                  tunnel: [w479] -> w447
                  tunnel: w456 -> [w478]
                  tunnel: [w482] -> w455
                  tunnel: [w477] -> w454
                  tunnel: [w476] -> w448
                  tunnel: w438 -> [w474]
                  tunnel: w437 -> [w473]
                  tunnel: [w503] -> w436
                  tunnel: w455 -> [w504]
                  tunnel: w454 -> [w502]
                  frame #0 {
                    n105 = call-poly <instrlib>:"Read.vi"("error in (no error)"=w459, "VISA resource name"=w460) -> ("error out"=w465:errorcluster, "Parameter Values"=w464:T10, "VISA resource name out"=w466:refnum<visa-resource-name>)  [unwired: 7 in]
                    n106 = Unbundle(w464) -> ("X-Value"=w463:dbl, "R-Value"=w462:dbl, "Theta-Value"=w461:dbl)  [unwired: 8 out]
                    "X-Value" <- w463
                    "Theta-Value" <- w461
                    "R-Value" <- w462
                  }
                  frame #1 {
                    n107 = call-poly <instrlib>:"Read.vi"("VISA resource name"=w469, "error in (no error)"=w468) -> ("Voltage"=w467:sgl, "VISA resource name out"=w472:refnum<visa-resource-name>, "Current"=w470:sgl, "error out"=w471:errorcluster)  [unwired: 7 in, 3 out]
                    "Voltage #1" <- w467
                    "Leakage Current #1" <- w470
                  }
                  frame #2 {
                    n108 = local read "Keithley #1 Ramp"() -> (w475:bool)
                    n109 = case shown="True" w475 {
                      tunnel: [w484 w501] -> w482
                      tunnel: w481 -> [w486 w500]
                      tunnel: w480 -> [w485 w499]
                      tunnel: [w485 w498] -> w479
                      tunnel: [w486 w497] -> w476
                      tunnel: w478 -> [_ w496]
                      tunnel: [FALSE ("END?") w495] -> w477
                      tunnel: w474 -> [_ w493]
                      tunnel: w473 -> [w484 w487]
                      frame False {
                      }
                      frame True {
                        n110 = Unbundle(w493) -> ("Keithley #1 Vg Init. (V)"=w492:dbl, "Keithley #1 Vg Max (V)"=w491:dbl, "Keithley #1 Vg Min (V)"=w490:dbl, "Keithley #1 Vg Step (V)"=w489:dbl, "Keith#1 Comp. Lvl"=w488:dbl)  [unwired: 4 out]
                        n111 = call "Keithley_Iterator.vi"("VISA resource name"=w500, "High Voltage"=w491, "Low Voltage"=w490, "Initial Voltage"=w492, "Iteration Input"=w487, "Current Voltage"=w496, "error in (no error)"=w499, "Voltage Step"=w489, "Compliance  Level (0.1)"=w488) -> ("VISA resource name out"=w497:refnum<visa-resource-name>, "Iteration Output"=w501:i32, "END?"=w495:bool, "error out"=w498:errorcluster)  [unwired: 2 in, 1 out]
                        n112 = property on="Keithley #1 Ramp" class="Bool (strict)"("DisabledEnum"=T9."Disabled and Grayed Out" ("Disabled")) -> ()  [unwired: 2 in, 2 out]
                      }
                    }
                  }
                  frame #3 {
                    n113 = case shown="True" w502 {
                      tunnel: w504 -> [w505 _]
                      tunnel: [w505 0 ("Iteration Output")] -> w503
                      frame False {
                      }
                      frame True {
                        # "Reset Iterator"
                        n114 = local write "Keithley #1 Ramp"(FALSE ("Keithley #1 Ramp")) -> ()
                        n115 = property on="Keithley #1 Ramp" class="Bool (strict)"("DisabledEnum"=T9."Enabled" ("Disabled")) -> ()  [unwired: 2 in, 2 out]
                      }
                    }
                  }
                }
                n116 = Bundle("Voltage"=w444, "Current"=w443, "X-Value"=w442, "R-Value"=w441, "Theta-Value"=w440) -> (w439:T8)  [unwired: 1 in]
                n117 = Bundle(cluster=w438, "VISA resource name out"=w448, "error out"=w447, "VISA resource name out"=w446, "error out"=w445) -> (w453:T3)  [unwired: 5 in]
              }
            }
          }
          frame #1 {
            # "Keithley & SR #2"
            n118 = case shown="True" w512 {
              tunnel: [w517 w535] -> w514
              tunnel: w513 -> [w517 w519]
              tunnel: [T8 {"Voltage"=0.0, "Current"=0.0, "X-Value"=0.0, "R-Value"=0.0, "Theta-Value"=0.0} w521] -> w511
              tunnel: w510 -> [w515 w520]
              tunnel: [w515 w518] -> w509
              frame False {
              }
              frame True {
                n119 = Unbundle(w519) -> ("VISA resource name out"=w528:refnum<visa-resource-name>, "error out"=w527:errorcluster, "VISA resource name out"=w530:refnum<visa-resource-name>, "error out"=w529:errorcluster)  [unwired: 5 out]
                n120 = flat-sequence {
                  tunnel: [w548] -> w534
                  tunnel: [w547] -> w533
                  tunnel: [w545] -> w524
                  tunnel: [w544] -> w523
                  tunnel: [w543] -> w522
                  tunnel: w530 -> [w542]
                  tunnel: w529 -> [w541]
                  tunnel: [w554] -> w540
                  tunnel: [w553] -> w539
                  tunnel: [w551] -> w538
                  tunnel: [w552] -> w525
                  tunnel: [w551] -> w526
                  tunnel: w528 -> [w550]
                  tunnel: w527 -> [w549]
                  tunnel: w540 -> [w563]
                  tunnel: w539 -> [w562]
                  tunnel: [w561] -> w531
                  tunnel: [w560] -> w532
                  tunnel: w538 -> [w559]
                  tunnel: [w564] -> w537
                  tunnel: [w558] -> w536
                  tunnel: w520 -> [w556]
                  tunnel: w519 -> [w555]
                  tunnel: [w585] -> w518
                  tunnel: w537 -> [w586]
                  tunnel: w536 -> [w584]
                  frame #0 {
                    n121 = call-poly <instrlib>:"Read.vi"("error in (no error)"=w541, "VISA resource name"=w542) -> ("error out"=w547:errorcluster, "Parameter Values"=w546:T10, "VISA resource name out"=w548:refnum<visa-resource-name>)  [unwired: 7 in]
                    n122 = Unbundle(w546) -> ("X-Value"=w545:dbl, "R-Value"=w544:dbl, "Theta-Value"=w543:dbl)  [unwired: 8 out]
                    "X-Value 2" <- w545
                    "Theta-Value 2" <- w543
                    "R-Value 2" <- w544
                  }
                  frame #1 {
                    n123 = call-poly <instrlib>:"Read.vi"("VISA resource name"=w550, "error in (no error)"=w549) -> ("Voltage"=w551:sgl, "VISA resource name out"=w554:refnum<visa-resource-name>, "Current"=w552:sgl, "error out"=w553:errorcluster)  [unwired: 7 in, 3 out]
                    "Voltage #2" <- w551
                    "Leakage Current #2" <- w552
                  }
                  frame #2 {
                    n124 = local read "Keithley #2 Ramp"() -> (w557:bool)
                    n125 = case shown="True" w557 {
                      tunnel: [w566 w583] -> w564
                      tunnel: w563 -> [w568 w582]
                      tunnel: w562 -> [w567 w581]
                      tunnel: [w567 w580] -> w561
                      tunnel: [w568 w579] -> w560
                      tunnel: w559 -> [_ w578]
                      tunnel: [FALSE ("END?") w577] -> w558
                      tunnel: w556 -> [w566 w575]
                      tunnel: w555 -> [_ w574]
                      frame False {
                      }
                      frame True {
                        n126 = Unbundle(w574) -> ("Keithley #2 Vg Init. (V)"=w573:dbl, "Keithley #2 Vg Max (V)"=w572:dbl, "Keithley #2 Vg Min (V)"=w571:dbl, "Keithley #2 Vg Step (V)"=w570:dbl, "Keith#2 Comp. Lvl"=w569:dbl)  [unwired: 4 out]
                        n127 = call "Keithley_Iterator.vi"("VISA resource name"=w582, "High Voltage"=w572, "Low Voltage"=w571, "Initial Voltage"=w573, "Iteration Input"=w575, "Current Voltage"=w578, "error in (no error)"=w581, "Voltage Step"=w570, "Compliance  Level (0.1)"=w569) -> ("VISA resource name out"=w579:refnum<visa-resource-name>, "Iteration Output"=w583:i32, "END?"=w577:bool, "error out"=w580:errorcluster)  [unwired: 2 in, 1 out]
                        n128 = property on="Keithley #2 Ramp" class="Bool (strict)"("DisabledEnum"=T9."Disabled and Grayed Out" ("Disabled")) -> ()  [unwired: 2 in, 2 out]
                      }
                    }
                  }
                  frame #3 {
                    n129 = case shown="True" w584 {
                      tunnel: w586 -> [w587 _]
                      tunnel: [w587 0 ("Iteration Output")] -> w585
                      frame False {
                      }
                      frame True {
                        # "Reset Iterator"
                        n130 = local write "Keithley #2 Ramp"(FALSE ("Keithley #1 Ramp")) -> ()
                        n131 = property on="Keithley #2 Ramp" class="Bool (strict)"("DisabledEnum"=T9."Enabled" ("Disabled")) -> ()  [unwired: 2 in, 2 out]
                      }
                    }
                  }
                }
                n132 = Bundle("Voltage"=w526, "Current"=w525, "X-Value"=w524, "R-Value"=w523, "Theta-Value"=w522) -> (w521:T8)  [unwired: 1 in]
                n133 = Bundle(cluster=w519, "VISA resource name out"=w532, "error out"=w531, "VISA resource name out"=w534, "error out"=w533) -> (w535:T5)  [unwired: 5 in]
              }
            }
          }
          frame #2 {
            # "Keithley & SR #3"
            n134 = case shown="True" w594 {
              tunnel: [w599 w617] -> w596
              tunnel: w595 -> [w599 w602]
              tunnel: [T8 {"Voltage"=0.0, "Current"=0.0, "X-Value"=0.0, "R-Value"=0.0, "Theta-Value"=0.0} w603] -> w593
              tunnel: w592 -> [w597 w601]
              tunnel: [w597 w600] -> w591
              frame False {
              }
              frame True {
                n135 = Unbundle(w602) -> ("VISA resource name out"=w616:refnum<visa-resource-name>, "error out"=w615:errorcluster, "VISA resource name out"=w614:refnum<visa-resource-name>, "error out"=w613:errorcluster)  [unwired: 5 out]
                n136 = flat-sequence {
                  tunnel: [w630] -> w612
                  tunnel: [w629] -> w611
                  tunnel: [w627] -> w606
                  tunnel: [w626] -> w605
                  tunnel: [w625] -> w604
                  tunnel: w614 -> [w624]
                  tunnel: w613 -> [w623]
                  tunnel: [w636] -> w622
                  tunnel: [w635] -> w621
                  tunnel: [w633] -> w620
                  tunnel: [w634] -> w607
                  tunnel: [w633] -> w608
                  tunnel: w616 -> [w632]
                  tunnel: w615 -> [w631]
                  tunnel: w622 -> [w645]
                  tunnel: w621 -> [w644]
                  tunnel: [w643] -> w609
                  tunnel: [w642] -> w610
                  tunnel: w620 -> [w641]
                  tunnel: [w646] -> w619
                  tunnel: [w640] -> w618
                  tunnel: w602 -> [w638]
                  tunnel: w601 -> [w637]
                  tunnel: [w667] -> w600
                  tunnel: w619 -> [w668]
                  tunnel: w618 -> [w666]
                  frame #0 {
                    n137 = call-poly <instrlib>:"Read.vi"("error in (no error)"=w623, "VISA resource name"=w624) -> ("error out"=w629:errorcluster, "Parameter Values"=w628:T10, "VISA resource name out"=w630:refnum<visa-resource-name>)  [unwired: 7 in]
                    n138 = Unbundle(w628) -> ("X-Value"=w627:dbl, "R-Value"=w626:dbl, "Theta-Value"=w625:dbl)  [unwired: 8 out]
                    "X-Value 3" <- w627
                    "Theta-Value 3" <- w625
                    "R-Value 3" <- w626
                  }
                  frame #1 {
                    n139 = call-poly <instrlib>:"Read.vi"("VISA resource name"=w632, "error in (no error)"=w631) -> ("Voltage"=w633:sgl, "VISA resource name out"=w636:refnum<visa-resource-name>, "Current"=w634:sgl, "error out"=w635:errorcluster)  [unwired: 7 in, 3 out]
                    "Voltage #3" <- w633
                    "Leakage Current #3" <- w634
                  }
                  frame #2 {
                    n140 = local read "Keithley #3 Ramp"() -> (w639:bool)
                    n141 = case shown="True" w639 {
                      tunnel: [w648 w665] -> w646
                      tunnel: w645 -> [w650 w664]
                      tunnel: w644 -> [w649 w663]
                      tunnel: [w649 w662] -> w643
                      tunnel: [w650 w661] -> w642
                      tunnel: w641 -> [_ w660]
                      tunnel: [FALSE ("END?") w659] -> w640
                      tunnel: w638 -> [_ w657]
                      tunnel: w637 -> [w648 w656]
                      frame False {
                      }
                      frame True {
                        n142 = Unbundle(w657) -> ("Keithley #3 Vg Init. (V)"=w655:dbl, "Keithley #3 Vg Max (V)"=w654:dbl, "Keithley #3 Vg Min (V)"=w653:dbl, "Keithley #3 Vg Step (V)"=w652:dbl, "Keith#3 Comp. Lvl"=w651:dbl)  [unwired: 4 out]
                        n143 = call "Keithley_Iterator.vi"("VISA resource name"=w664, "High Voltage"=w654, "Low Voltage"=w653, "Initial Voltage"=w655, "Iteration Input"=w656, "Current Voltage"=w660, "error in (no error)"=w663, "Voltage Step"=w652, "Compliance  Level (0.1)"=w651) -> ("VISA resource name out"=w661:refnum<visa-resource-name>, "Iteration Output"=w665:i32, "END?"=w659:bool, "error out"=w662:errorcluster)  [unwired: 2 in, 1 out]
                        n144 = property on="Keithley #3 Ramp" class="Bool (strict)"("DisabledEnum"=T9."Disabled and Grayed Out" ("Disabled")) -> ()  [unwired: 2 in, 2 out]
                      }
                    }
                  }
                  frame #3 {
                    n145 = case shown="True" w666 {
                      tunnel: w668 -> [w669 _]
                      tunnel: [w669 0 ("Iteration Output")] -> w667
                      frame False {
                      }
                      frame True {
                        # "Reset Iterator"
                        n146 = local write "Keithley #3 Ramp"(FALSE ("Keithley #1 Ramp")) -> ()
                        n147 = property on="Keithley #3 Ramp" class="Bool (strict)"("DisabledEnum"=T9."Enabled" ("Disabled")) -> ()  [unwired: 2 in, 2 out]
                      }
                    }
                  }
                }
                n148 = Bundle("Voltage"=w608, "Current"=w607, "X-Value"=w606, "R-Value"=w605, "Theta-Value"=w604) -> (w603:T8)  [unwired: 1 in]
                n149 = Bundle(cluster=w602, "VISA resource name out"=w610, "error out"=w609, "VISA resource name out"=w612, "error out"=w611) -> (w617:T6)  [unwired: 5 in]
              }
            }
          }
        }
      }
      frame #2 {
        w726 = "%.12f" ("format string")
        w723 = "\t"
        # "Theta"
        # "X"
        # "Current"
        # "Voltage"
        # "Field"
        # "Temperature"
        # "Write #3"
        # "Write #2"
        # "Write #1"
        # "Conclusion"
        n150 = Unbundle(w734) -> ("System #1 Enabled/Disabled"=w733:bool, "System #2 Enabled/Disabled"=w728:bool, "System #3 Enabled/Disabled"=w727:bool)
        n151 = Unbundle(w731) -> ("Temperature"=w711:dbl, "Field"=w709:dbl)
        n152 = local write "Measuring"(FALSE ("Measuring")) -> ()
        n153 = Format Into String(format string=w726, w711) -> (resulting string=w725:string)  [unwired: 2 in, 1 out]
        n154 = Format Into String(format string=w726, w709) -> (resulting string=w724:string)  [unwired: 2 in, 1 out]
        n155 = Concatenate Strings(w725, w723, w724) -> (w722:string)
        n156 = case shown="True" w733 {
          tunnel: w732 -> [_ w829]
          tunnel: w726 -> [_ w827]
          tunnel: w723 -> [_ w818]
          tunnel: w722 -> [w808 w819]
          tunnel: [w808 w820] -> w721
          tunnel: dbl[] [] ("array") -> [w807 w813]
          tunnel: [w807 w812] -> w699
          tunnel: [w807 w811] -> w698
          tunnel: [w807 w810] -> w697
          tunnel: [w807 w809] -> w696
          frame False {
          }
          frame True {
            n157 = Unbundle(w829) -> ("Voltage"=w817:sgl, "Current"=w816:sgl, "X-Value"=w815:dbl, "R-Value"=w828:dbl, "Theta-Value"=w814:dbl)
            n158 = Format Into String(format string=w827, w817) -> (resulting string=w826:string)  [unwired: 2 in, 1 out]
            n159 = Format Into String(format string=w827, w816) -> (resulting string=w825:string)  [unwired: 2 in, 1 out]
            n160 = Format Into String(format string=w827, w815) -> (resulting string=w824:string)  [unwired: 2 in, 1 out]
            n161 = Format Into String(format string=w827, w814) -> (resulting string=w822:string)  [unwired: 2 in, 1 out]
            n162 = Insert Into Array(array=w813, new element=w816) -> (w811:dbl[])  [unwired: 1 in]
            n163 = Insert Into Array(array=w813, new element=w817) -> (w812:dbl[])  [unwired: 1 in]
            n164 = Insert Into Array(array=w813, new element=w814) -> (w809:dbl[])  [unwired: 1 in]
            n165 = Insert Into Array(array=w813, new element=w815) -> (w810:dbl[])  [unwired: 1 in]
            n166 = Format Into String(format string=w827, initial string=w824, w828) -> (resulting string=w823:string)  [unwired: 1 in, 1 out]
            n167 = Concatenate Strings(w826, w818, w825, w818, w824, w818, w823, w818, w822) -> (w821:string)
            n168 = Concatenate Strings(w819, w818, w821) -> (w820:string)
          }
        }
        n169 = Unbundle(w708) -> ("array"=w712:dbl[], "array"=w710:dbl[])
        n170 = case shown="True" w728 {
          tunnel: w730 -> [_ w806]
          tunnel: w726 -> [_ w804]
          tunnel: w723 -> [_ w797]
          tunnel: w721 -> [w782 w798]
          tunnel: [w782 w795] -> w720
          tunnel: w699 -> [w781 w794]
          tunnel: w698 -> [w780 w793]
          tunnel: w697 -> [w779 w792]
          tunnel: w696 -> [w778 w791]
          tunnel: [w781 w786] -> w695
          tunnel: [w780 w785] -> w694
          tunnel: [w779 w784] -> w693
          tunnel: [w778 w783] -> w692
          frame False {
          }
          frame True {
            n171 = Unbundle(w806) -> ("Voltage"=w790:sgl, "Current"=w789:sgl, "X-Value"=w788:dbl, "R-Value"=w805:dbl, "Theta-Value"=w787:dbl)
            n172 = Format Into String(format string=w804, w790) -> (resulting string=w803:string)  [unwired: 2 in, 1 out]
            n173 = Format Into String(format string=w804, w789) -> (resulting string=w802:string)  [unwired: 2 in, 1 out]
            n174 = Format Into String(format string=w804, w788) -> (resulting string=w801:string)  [unwired: 2 in, 1 out]
            n175 = Format Into String(format string=w804, w787) -> (resulting string=w799:string)  [unwired: 2 in, 1 out]
            n176 = Insert Into Array(array=w793, new element=w789) -> (w785:dbl[])  [unwired: 1 in]
            n177 = Insert Into Array(array=w794, new element=w790) -> (w786:dbl[])  [unwired: 1 in]
            n178 = Insert Into Array(array=w791, new element=w787) -> (w783:dbl[])  [unwired: 1 in]
            n179 = Insert Into Array(array=w792, new element=w788) -> (w784:dbl[])  [unwired: 1 in]
            n180 = Format Into String(format string=w804, initial string=w801, w805) -> (resulting string=w800:string)  [unwired: 1 in, 1 out]
            n181 = Concatenate Strings(w803, w797, w802, w797, w801, w797, w800, w797, w799) -> (w796:string)
            n182 = Concatenate Strings(w798, w797, w796) -> (w795:string)
          }
        }
        n183 = case shown="True" w727 {
          tunnel: w729 -> [_ w777]
          tunnel: w726 -> [_ w775]
          tunnel: w723 -> [_ w768]
          tunnel: w720 -> [w753 w767]
          tunnel: [w753 w766] -> w719
          tunnel: w695 -> [w752 w765]
          tunnel: w694 -> [w751 w764]
          tunnel: w693 -> [w750 w763]
          tunnel: w692 -> [w749 w762]
          tunnel: [w752 w757] -> w691
          tunnel: [w751 w756] -> w690
          tunnel: [w750 w755] -> w689
          tunnel: [w749 w754] -> w688
          frame False {
          }
          frame True {
            n184 = Unbundle(w777) -> ("Voltage"=w761:sgl, "Current"=w760:sgl, "X-Value"=w759:dbl, "R-Value"=w776:dbl, "Theta-Value"=w758:dbl)
            n185 = Format Into String(format string=w775, w761) -> (resulting string=w774:string)  [unwired: 2 in, 1 out]
            n186 = Format Into String(format string=w775, w760) -> (resulting string=w773:string)  [unwired: 2 in, 1 out]
            n187 = Format Into String(format string=w775, w759) -> (resulting string=w772:string)  [unwired: 2 in, 1 out]
            n188 = Format Into String(format string=w775, w758) -> (resulting string=w770:string)  [unwired: 2 in, 1 out]
            n189 = Insert Into Array(array=w764, new element=w760) -> (w756:dbl[])  [unwired: 1 in]
            n190 = Insert Into Array(array=w765, new element=w761) -> (w757:dbl[])  [unwired: 1 in]
            n191 = Insert Into Array(array=w762, new element=w758) -> (w754:dbl[])  [unwired: 1 in]
            n192 = Insert Into Array(array=w763, new element=w759) -> (w755:dbl[])  [unwired: 1 in]
            n193 = Format Into String(format string=w775, initial string=w772, w776) -> (resulting string=w771:string)  [unwired: 1 in, 1 out]
            n194 = Concatenate Strings(w774, w768, w773, w768, w772, w768, w771, w768, w770) -> (w769:string)
            n195 = Concatenate Strings(w767, w768, w769) -> (w766:string)
          }
        }
        n196 = Unbundle(w702) -> ("array"=w703:dbl[][], "array"=w704:dbl[][], "array"=w705:dbl[][], "array"=w706:dbl[][])
        n197 = Build Array (concatenate)(w704, w690) -> (w686:dbl[][])
        n198 = Build Array (concatenate)(w703, w691) -> (w687:dbl[][])
        n199 = Build Array (concatenate)(w706, w688) -> (w684:dbl[][])
        n200 = Build Array (concatenate)(w705, w689) -> (w685:dbl[][])
        n201 = Concatenate Strings(w719, "\r\n") -> (w717:string)
        n202 = Transpose 2D Array(2D array=w686) -> (transposed array=w682:dbl[][])
        n203 = Transpose 2D Array(2D array=w687) -> (transposed array=w683:dbl[][])
        n204 = Transpose 2D Array(2D array=w684) -> (transposed array=w678:dbl[][])
        n205 = Bundle(w687, w686, w685, w684) -> (w701:cluster{dbl[][], dbl[][], dbl[][], dbl[][]})  [unwired: 1 in]
        n206 = Transpose 2D Array(2D array=w685) -> (transposed array=w680:dbl[][])
        n207 = Build Array (concatenate)(w710, w709) -> (w675:dbl[])
        n208 = Build Array (concatenate)(w712, w711) -> (w676:dbl[])
        n209 = Write to Text File(file (use dialog)=w716, text=w717, error in=w714) -> (refnum out=w715:refnum<file>, error out=w713:errorcluster)  [unwired: 1 in, 1 out]
        n210 = for {
          tunnel: w683 -> [w744] mode=indexing
          tunnel: w682 -> [w748] mode=indexing
          tunnel: [w747] -> w681 mode=indexing
          tunnel: w680 -> [w740] mode=indexing
          tunnel: [w746] -> w679 mode=indexing
          tunnel: w678 -> [w745] mode=indexing
          tunnel: [w743] -> w677 mode=indexing
          tunnel: w676 -> [w742]
          tunnel: w675 -> [w741]
          tunnel: [w739] -> w674 mode=indexing
          tunnel: [w738] -> w673 mode=indexing
          n211 = Bundle(w744, w748) -> (w747:cluster{dbl[], dbl[]})  [unwired: 1 in]
          n212 = Bundle(w744, w740) -> (w746:cluster{dbl[], dbl[]})  [unwired: 1 in]
          n213 = Bundle(w744, w745) -> (w743:cluster{dbl[], dbl[]})  [unwired: 1 in]
          n214 = Bundle(w741, w740) -> (w739:cluster{dbl[], dbl[]})  [unwired: 1 in]
          n215 = Bundle(w742, w740) -> (w738:cluster{dbl[], dbl[]})  [unwired: 1 in]
        }
        "Signal-T" <- w673
        "Leak-Vg" <- w681
        "Phase-Vg" <- w677
        "Signal-B" <- w674
        "Signal-Vg" <- w679
        n216 = Bundle(w676, w675) -> (w707:cluster{dbl[], dbl[]})  [unwired: 1 in]
      }
    }
    n217 = Wait (ms)(milliseconds to wait=u32 1000) -> ()  [unwired: 1 out]
  }
  n218 = Close File(refnum=w22, error in=w21) -> (error out=w26:errorcluster)  [unwired: 1 out]
  n219 = call <vilib>:"Simple Error Handler.vi"("error in (no error)"=w26) -> ()  [unwired: 4 in, 5 out]
  n220 = Close Reference(reference=w23, error in (no error)=w24) -> ()  [unwired: 1 out]
  n221 = Unbundle(w13) -> ("System #1 Enabled/Disabled"=w12:bool, "System #2 Enabled/Disabled"=w11:bool, "System #3 Enabled/Disabled"=w10:bool)
  n222 = case shown="True" w11 {
    tunnel: w3 -> [_ w834]
    frame False {
    }
    frame True {
      n223 = Unbundle(w834) -> ("VISA resource name out"=w831:refnum<visa-resource-name>, "error out"=w830:errorcluster, "VISA resource name out"=w833:refnum<visa-resource-name>, "error out"=w832:errorcluster)  [unwired: 5 out]
      n224 = call <instrlib>:"Close.vi"("error in (no error)"=w832, "VISA resource name"=w833) -> ("error out"=w835:errorcluster)  [unwired: 9 in]
      n225 = call <instrlib>:"Close.vi"("error in (no error)"=w830, "VISA resource name"=w831) -> ("error out"=w836:errorcluster)  [unwired: 9 in]
      n226 = call <vilib>:"Simple Error Handler.vi"("error in (no error)"=w835) -> ()  [unwired: 4 in, 5 out]
      n227 = call <vilib>:"Simple Error Handler.vi"("error in (no error)"=w836) -> ()  [unwired: 4 in, 5 out]
    }
  }
  n228 = case shown="True" w12 {
    tunnel: w4 -> [_ w841]
    frame False {
    }
    frame True {
      n229 = Unbundle(w841) -> ("VISA resource name out"=w840:refnum<visa-resource-name>, "error out"=w839:errorcluster, "VISA resource name out"=w838:refnum<visa-resource-name>, "error out"=w837:errorcluster)  [unwired: 5 out]
      n230 = call <instrlib>:"Close.vi"("error in (no error)"=w837, "VISA resource name"=w838) -> ("error out"=w842:errorcluster)  [unwired: 9 in]
      n231 = call <instrlib>:"Close.vi"("error in (no error)"=w839, "VISA resource name"=w840) -> ("error out"=w843:errorcluster)  [unwired: 9 in]
      n232 = call <vilib>:"Simple Error Handler.vi"("error in (no error)"=w842) -> ()  [unwired: 4 in, 5 out]
      n233 = call <vilib>:"Simple Error Handler.vi"("error in (no error)"=w843) -> ()  [unwired: 4 in, 5 out]
    }
  }
  n234 = case shown="True" w10 {
    tunnel: w2 -> [_ w848]
    frame False {
    }
    frame True {
      n235 = Unbundle(w848) -> ("VISA resource name out"=w847:refnum<visa-resource-name>, "error out"=w846:errorcluster, "VISA resource name out"=w845:refnum<visa-resource-name>, "error out"=w844:errorcluster)  [unwired: 5 out]
      n236 = call <instrlib>:"Close.vi"("error in (no error)"=w844, "VISA resource name"=w845) -> ("error out"=w849:errorcluster)  [unwired: 9 in]
      n237 = call <instrlib>:"Close.vi"("error in (no error)"=w846, "VISA resource name"=w847) -> ("error out"=w850:errorcluster)  [unwired: 9 in]
      n238 = call <vilib>:"Simple Error Handler.vi"("error in (no error)"=w849) -> ()  [unwired: 4 in, 5 out]
      n239 = call <vilib>:"Simple Error Handler.vi"("error in (no error)"=w850) -> ()  [unwired: 4 in, 5 out]
    }
  }
  "Measuring" <- FALSE ("Measuring")
